vi "CRYScope-FFT.vi"(0 "Mode":u32(ring) items=["Time", "Spectrum"], 1 "Signal Path":i32(ring), 2 "Averages":i32=1 min=1, 3 "Time(sec)":dbl=0.05 min=0.05 max=10.0 step=0.05 format="%#.6p", 4 "Start":bool, 6 "Snap":bool, 7 "Hardware":string, 8 "Lin/Exp":i32(slide), 9 "Execution control":T6={"interactive"=TRUE, "displayed"=TRUE, "in a seq"=FALSE}, 10 "Manual":bool=TRUE, 11 "Calibration":string, 12 "Power/Complex":i32(slide)) -> (14 "Data cluster":T4, 16 "Avg. Complete":i32, 17 "Selected Signal Path":string, 18 "scope-fft setup Out":string="%#_6p", 19 "Canceled":bool)   [LabVIEW 2013]
uses:
  Typedef Control/CRYWaveform Cluster.ctl
  Typedef Control/CRYCalibration 2DCluster.ctl
  Typedef Control/CRYCalibration Cluster.ctl
  Typedef Control/CRYData Cluster.ctl
  Typedef Control/CRYHardware Channel Info.ctl
  SubVI/CRYMisc vis settings global.vi
  CRYMainGlobal.vi
  Calibration/SubVI/CRYCal Global.vi
  Task Sequence/CRYProject Run Control Global.vi
  <vilib>/Analysis/NI_AALPro.lvlib
  CRYSound.dll
panel:
  in  "Buf Cnt":i32
  in  "isMain":bool
  in  "Rcv Idx":u16
  in  "start_flg":u8
  in  "Remain Data":i32[](array[numeric])
  out "Asio OCI":u32
  in  "Device Name":string
  in  "ASIO_Inited":bool
  in  "Audio Driver":u16
  out "Max Level":dbl
  out "Load Test":bool
  out "Configure Data":string
  out "Set Configure":bool
  out "Calibration All Cluster":T1={"Calibration"={"Calibration Step Name"="", "Device"="", "Correction Curve Name"="", "Equalization Curve Name"="", "Sensitivity Curve Name"="", "Corr Folder and File"="", "EQ Folder and File"="", "Sens Folder and File"="", "Corr Step size"=0, "EQ Step size"=0, "Input"=FALSE, "Last Cal Date (sec)"=timestamp(0 s since 1904-01-01), "Cha Name"="", "Corr Curve Found"=FALSE, "EQ Curve Found"=FALSE, "Sens Curve Found"=FALSE, "Signal Type"="", "Calibrated Device"="", "Hz"=0}, "Corr Curve"={"Name"="", "Curve"=[], "X data"=1, "Y data"=1, "Z data"=1, "X axis"=0, "Y axis"=1, "Z axis"=1, "X unit"="", "Y unit"="", "Z unit"="deg.", "X dB ref"=1.0, "Y dB ref"=1.0, "Z dB ref"=1.0, "single val"=FALSE, "protected"=FALSE, "display X"=FALSE, "display Y"=TRUE, "display Z"=TRUE, "Test Info"="", "Step No."=0, "Plot Settings"={"Color"=0, "Interpolation"=0, "Point Style"=0, "Line Style"=0, "Point Color"=0, "Line Width"=0, "Bar Plot Style"=0, "Fill To"=0}, "AutoProtect"=FALSE}, "EQ Curve"={"Name"="", "Curve"=[], "X data"=1, "Y data"=1, "Z data"=1, "X axis"=0, "Y axis"=1, "Z axis"=1, "X unit"="Hz", "Y unit"="", "Z unit"="deg.", "X dB ref"=1.0, "Y dB ref"=1.0, "Z dB ref"=1.0, "single val"=FALSE, "protected"=FALSE, "display X"=TRUE, "display Y"=TRUE, "display Z"=TRUE, "Test Info"="", "Step No."=0, "Plot Settings"={"Color"=0, "Interpolation"=0, "Point Style"=0, "Line Style"=0, "Point Color"=0, "Line Width"=0, "Bar Plot Style"=0, "Fill To"=0}, "AutoProtect"=FALSE}, "Sens Curve"={"Name"="", "Curve"=[], "X data"=1, "Y data"=1, "Z data"=1, "X axis"=0, "Y axis"=1, "Z axis"=1, "X unit"="Hz", "Y unit"="", "Z unit"="deg.", "X dB ref"=1.0, "Y dB ref"=1.0, "Z dB ref"=1.0, "single val"=FALSE, "protected"=FALSE, "display X"=TRUE, "display Y"=TRUE, "display Z"=TRUE, "Test Info"="", "Step No."=0, "Plot Settings"={"Color"=0, "Interpolation"=0, "Point Style"=0, "Line Style"=0, "Point Color"=0, "Line Width"=0, "Bar Plot Style"=0, "Fill To"=0}, "AutoProtect"=FALSE}} {"Sens Curve"."Z data" items=["dB", "Lin"]; "Sens Curve"."X data" items=["dB", "Lin"]; "Sens Curve"."Y data" items=["dB", "Lin"]; "Sens Curve"."Z dB ref" format="%.1f"; "Sens Curve"."Z axis" items=["Log", "Lin"]; "Sens Curve"."X dB ref" format="%.1f"; "Sens Curve"."X axis" items=["Log", "Lin"]; "Sens Curve"."Y axis" items=["Log", "Lin"]; "Sens Curve"."Y dB ref" format="%.1f"; "Sens Curve"."Curve"."z" format="%.2f"; "Sens Curve"."Curve"."y" format="%.2f"; "Sens Curve"."Curve"."x" format="%.2f"; "EQ Curve"."Z data" items=["dB", "Lin"]; "EQ Curve"."X data" items=["dB", "Lin"]; "EQ Curve"."Y data" items=["dB", "Lin"]; "EQ Curve"."Z dB ref" format="%.1f"; "EQ Curve"."Z axis" items=["Log", "Lin"]; "EQ Curve"."X dB ref" format="%.1f"; "EQ Curve"."X axis" items=["Log", "Lin"]; "EQ Curve"."Y axis" items=["Log", "Lin"]; "EQ Curve"."Y dB ref" format="%.1f"; "EQ Curve"."Curve"."z" format="%.2f"; "EQ Curve"."Curve"."y" format="%.2f"; "EQ Curve"."Curve"."x" format="%.2f"; "Corr Curve"."Z data" items=["dB", "Lin"]; "Corr Curve"."X data" items=["dB", "Lin"]; "Corr Curve"."Y data" items=["dB", "Lin"]; "Corr Curve"."Z dB ref" format="%.1f"; "Corr Curve"."Z axis" items=["Log", "Lin"]; "Corr Curve"."X dB ref" format="%.1f"; "Corr Curve"."X axis" items=["Log", "Lin"]; "Corr Curve"."Y axis" items=["Log", "Lin"]; "Corr Curve"."Y dB ref" format="%.1f"; "Corr Curve"."Curve"."z" format="%.2f"; "Corr Curve"."Curve"."y" format="%.2f"; "Corr Curve"."Curve"."x" format="%.2f"; "Calibration"."EQ Step size" items=["R10", "R20", "R40", "R80", "User"]; "Calibration"."Corr Step size" items=["R10", "R20", "R40", "R80", "User"]}
  out "Est.Unit":string
  out "dB":dbl caption="Est.Level" format="%.3g"
  out "Cursor":bool
  out "initialized array":i32[](array[numeric])
  out "Menu":bool=TRUE
  out "StateOut":bool=TRUE
  out "VI nID":i32
  out "Title nID":i32
  in  "delta_Y":dbl
  in  "delta_X":dbl format="%#.3p"
  in  "delta_str":string
  out "rem buffer":i32[](array[numeric])
  out "dB Est.Level":dbl=33.979400086720375 format="%.2p"
  out "Channel In":u16
  in  "Waveform Cluster":T5={"Waveform"={"X0"=0.0, "dX"=0.0, "Y"=[]}, "X data"=1, "Y data"=1, "Y axis"=1, "X unit"="s", "Y unit"="s", "Y dB ref"=1.0, "display Y"=TRUE, "display X"=TRUE, "Overload?"=TRUE, "Test Info"="", "Step No."=0, "Name"="", "protected"=FALSE, "Sqc history"=[], "Signal Channel ID"=0, "Plot Settings"={"Color"=0, "Interpolation"=0, "Point Style"=0, "Line Style"=0, "Point Color"=0, "Line Width"=0, "Bar Plot Style"=0, "Fill To"=0}, "AutoProtect"=FALSE} {"Y dB ref" format="%.1f"; "Y axis" items=["Log", "Lin"]; "Y data" items=["dB", "Lin"]; "X data" items=["dB", "Lin"]}
  out "Triggered":bool
  out "AvgT":bool
  in  "Window":u16(ring) items=["None"=0, "Hanning"=1, "Hamming"=2, "Blackman-Harris"=3, "Exact Blackman"=4, "Blackman"=5, "Flat Top"=6, "4 Term B-Harris"=7, "7 Term B-Harris"=8, "Low Sidelobe"=9, "Blackman Nuttall"=11, "Triangle"=30, "Modified Bartlett-Hanning"=31, "Bohman"=32, "Parzen"=33, "Welch"=34, "Kaiser"=60, "Dolph-Chebyshev"=61, "Gaussian"=62]
  out "Spectrum graph":cluster{dbl, "df":dbl, "Spectrum":dbl[]}(graph)
  out "Buffer":u8(slide) scale=0.0..100.0
  out "Signal Graph":bool
  out "Averaging":bool
  out "Resolution":bool
  out "Input":bool
  out "Spectrum":bool
  out "Trigger":bool
  in  "taskID":u32
  out "Overload":bool
  in  "Slope":u32(slide) scale=0.0..1.0
  in  "Trigger Unit":u32(slide) scale=0.0..1.0
  out "Scale":bool
  in  "n points":i32=2048 caption="FFT lines" min=256 max=100000 step=256
  in  "Channels":u8=2
  out "Device In":u32
  in  "cont loop":bool=TRUE
  in  "Sensitivity":dbl=1.0 caption="V/unit" format="%.4f"
  in  "dB ref.":dbl=1.0 format="%.2f"
  in  "Y Unit":string
  in  "Y-axis":u16(ring) items=["dB", "Linear"]
  out "VMax In":dbl=10.0 format="%.3f"
  out "Bits":u32=16
  out "Sampling rate":u32=44100
  in  "close at end":bool
  out "THD":dbl max=10.0 format="%#_4p"
  in  "Harmonic":bool caption="Harmonic Cursor"
  in  "CalSpectrum":bool=TRUE caption="Calculate Spectrum"
  out "Hz":dbl caption="Est.Freq" format="%.1f"
  in  "Continue":bool
  in  "Correct":bool caption="Apply Correction"
  out "Real Time":u8(slide) scale=0.0..10.0
  out "Time graph":T7(graph)
  in  "dF(Hz)":dbl format="%#_6p"
  in  "dT(sec)":dbl format="%#_6p"
  in  "Spectral Lines":dbl min=256.0 format="%#_4p"
  in  "FreeRun":bool
  in  "Trigger Offset(sec)":dbl caption="Trigger Offset(s)" min=-0.05 max=0.05 format="%#_6p"
  in  "Trigger Level":dbl format="%#_5p"
  in  "Cancel":bool
  in  "Save":bool
  in  "OK":bool
  in  "A/M/M":i32(slide)
  in  "Trigger Path":u16(ring)
  in  "Weighting":u16(ring) items=["None", "A", "B", "C"]
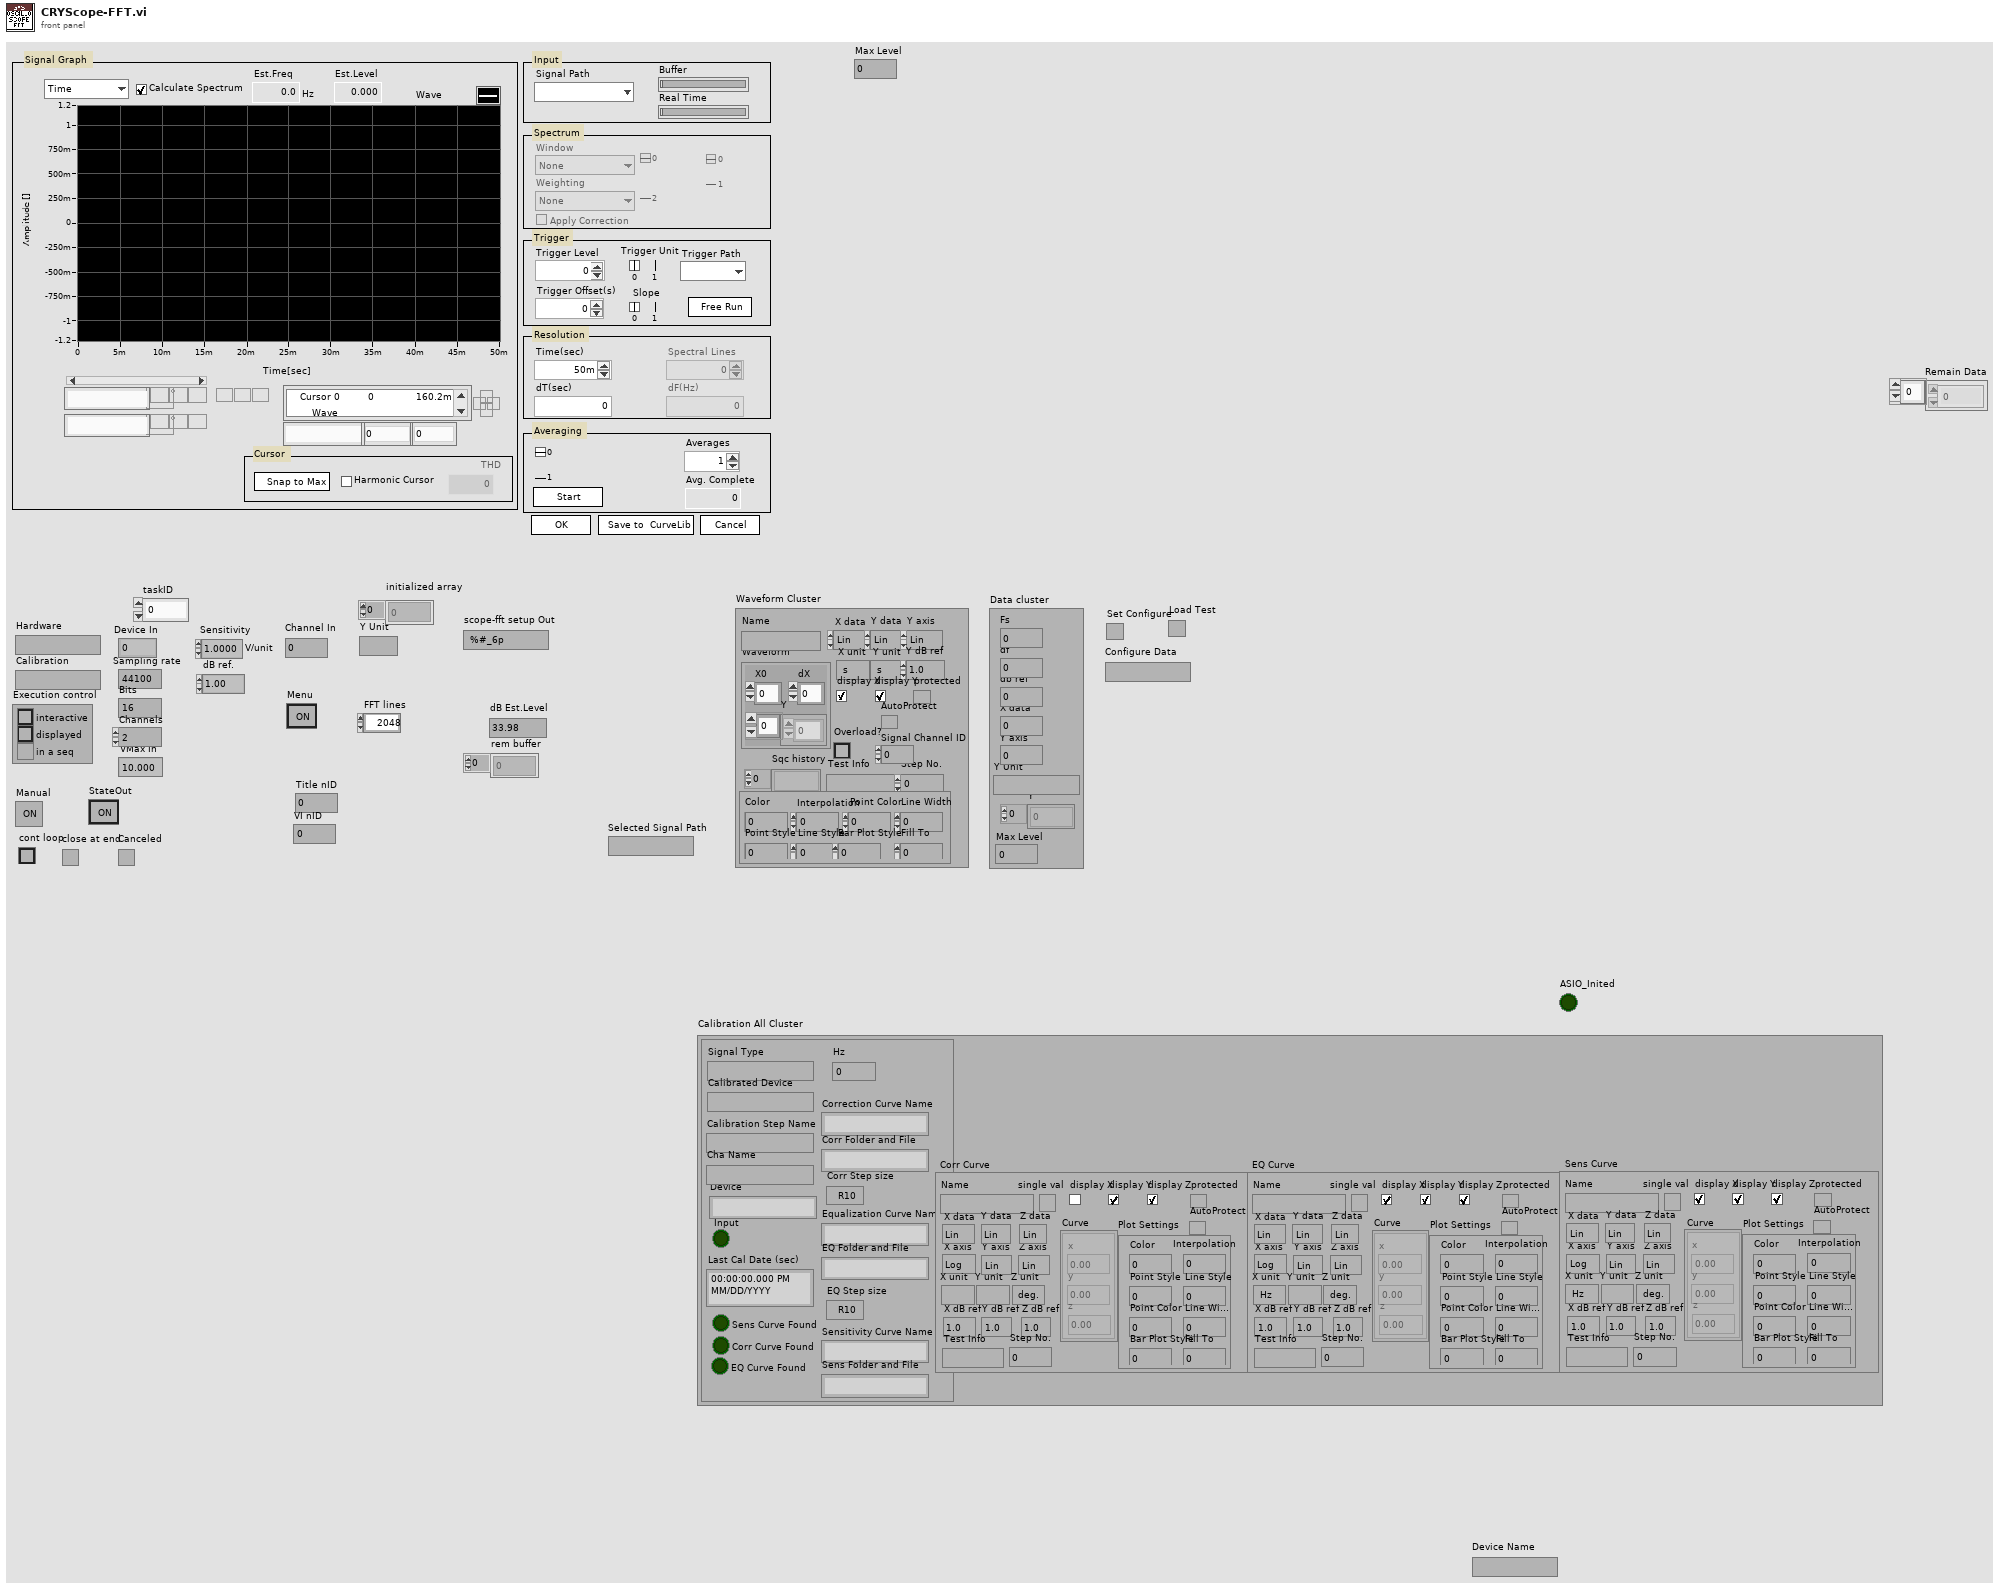
[diagram p1: front panel]
types:
  T1 = typedef "CRYCalibration 2DCluster.ctl" = cluster{"Calibration":T2, "Corr Curve":T3, "EQ Curve":T3, "Sens Curve":T3}
  T2 = typedef "CRYCalibration Cluster.ctl" = cluster{"Calibration Step Name":string, "Device":string, "Correction Curve Name":string, "Equalization Curve Name":string, "Sensitivity Curve Name":string, "Corr Folder and File":string, "EQ Folder and File":string, "Sens Folder and File":string, "Corr Step size":u16, "EQ Step size":u16, "Input":bool, "Last Cal Date (sec)":timestamp, "Cha Name":string, "Corr Curve Found":bool, "EQ Curve Found":bool, "Sens Curve Found":bool, "Signal Type":string, "Calibrated Device":string, "Hz":u32}
  T3 = typedef "CRYData Cluster.ctl" = cluster{"Name":string, "Curve":cluster{"x":dbl, "y":dbl, "z":dbl}[], "X data":u16, "Y data":u16, "Z data":u16, "X axis":u16, "Y axis":u16, "Z axis":u16, "X unit":string, "Y unit":string, "Z unit":string, "X dB ref":dbl, "Y dB ref":dbl, "Z dB ref":dbl, "single val":bool, "protected":bool, "display X":bool, "display Y":bool, "display Z":bool, "Test Info":string, "Step No.":i32, "Plot Settings":cluster{"Color":u32, "Interpolation":u8, "Point Style":u8, "Line Style":u8, "Point Color":u32, "Line Width":u8, "Bar Plot Style":u8, "Fill To":i16}, "AutoProtect":bool}
  T4 = cluster{"Fs":dbl, "df":dbl, "db ref":dbl, "X data":u16, "Y axis":u16, "Y Unit":string, "Y":dbl[], "Max Level":dbl}
  T5 = typedef "CRYWaveform Cluster.ctl" = cluster{"Waveform":cluster{"X0":dbl, "dX":dbl, "Y":sgl[]}, "X data":u16, "Y data":u16, "Y axis":u16, "X unit":string, "Y unit":string, "Y dB ref":dbl, "display Y":bool, "display X":bool, "Overload?":bool, "Test Info":string, "Step No.":i32, "Name":string, "protected":bool, "Sqc history":string[], "Signal Channel ID":i32, "Plot Settings":cluster{"Color":u32, "Interpolation":u8, "Point Style":u8, "Line Style":u8, "Point Color":u32, "Line Width":u8, "Bar Plot Style":u8, "Fill To":i16}, "AutoProtect":bool}
  T6 = cluster{"interactive":bool, "displayed":bool, "in a seq":bool}
  T7 = cluster{dbl, "dT(sec)":dbl, "Triggered signal":dbl[]}
  T8 = cluster{"window":i32, "n avgs":i32, "lin/exp avg":i32, "pwr/cplx avg":i32, "time (ms)":dbl, "fft lines":i32, "scope/fft mode":i32, "channel":i32, "trig. channel":i32, "Applay Correction":bool, "Time Display":string, "Freq. Weighting":string, "Ave/Max/Min":u16, "Trigger Level":dbl, "Trigger Unit":u16, "Trigger Time Offset":dbl, "Trigger Slope":u16, "Trigger/Free Run":bool, "continuous":bool, "Spectrum Display":string, "Calc FFT":bool, "Y-axis":string, "Channel String":string}
  T9 = enum32{"Invalid", "Default", "Floating", "Floating/Auto-Hide", "Modal"}
  T10 = cluster{"Weighting":u16, "Signal Path":i32, "Y-axis":u16, "Time(sec)":dbl, "Mode":u32, "Power/Complex":i32, "Harmonic":bool, "Trigger Level":dbl, "n points":i32, "Lin/Exp":i32, "Trigger Offset(sec)":dbl, "Trigger Unit":u32, "Averages":i32, "Start":bool, "Spectral Lines":dbl, "A/M/M":i32, "FreeRun":bool}
  T11 = typedef "CRYCalibration All Cluster.ctl" = cluster{"Calibration 2D":T1[], "Help":string, "Tab Value":i32, "Input Signal Type":string, "Output Signal Type":string}
  T12 = typedef "CRYScope-FFT.ctl" = cluster{"window":i32, "n avgs":i32, "lin/exp avg":i32, "pwr/cplx avg":i32, "time (ms)":dbl, "fft lines":i32, "scope/fft mode":i32, "channel":i32, "trig. channel":i32, "Applay Correction":bool, "Time Display":string, "Freq. Weighting":string, "Ave/Max/Min":u16, "Trigger Level":dbl, "Trigger Unit":u16, "Trigger Time Offset":dbl, "Trigger Slope":u16, "Trigger/Free Run":bool, "continuous":bool, "Spectrum Display":string, "Calc FFT":bool, "Y-axis":string, "Signal Type":string}
  T13 = typedef "CRYHardware Channel Info.ctl" = cluster{"ID":i32, "Name":string, "Digital":bool, "Input":bool, "Device Name":string, "Hardware Ch ID":u8, "Vmax (V)":dbl, "Latency (samples)":dbl, "Sampling Rate (Hz)":u32, "Bit Depth":u32, "Anti-aliasing Factor (%fs)":sgl, "DAQmx Channel":tag, "term config":i32, "Coupling":i32, "IEPE en":bool, "ASIOChannel Name":string, "Audio Driver":u16, "ASIOChannel Index":u8}
  T14 = enum32{"English", "Chinese", "Korean", "Japanese", "Russian", "Chinese traditional"}
  T15 = enum32{"Vrms", "Vpk", "Vrms^2", "Vpk^2", "Vrms/rtHz", "Vpk/rtHz", "Vrms^2/Hz", "Vpk^2/Hz"}
  T16 = cluster{"acquire":bool, "halt acq":bool, "cal factor":dbl, "n avgd":i32, "db-pr factor":dbl, "points":i32, "buffers":i32, "points chg":bool, "db ref":dbl, "df":dbl, "window constants":cluster{"eq noise BW":dbl, "coherent gain":dbl}, "cursor index":i32, "cursor x":dbl, "trig level":i32, "est freq":dbl, "est power":dbl, "update":bool, "autoscale":bool, "avg. complete":i32, "prebuffer":i32, "nextbuffer":i32, "addbuffs":i32, "Y-axis chg":bool, "Weight":cluster{dbl, dbl}[]}
  T17 = typedef "CRYStimulus Test Infor Cluster.ctl" = cluster{"Stimulus Type":string, "Signal Type":string, "In/Out":bool, "FAPS":cluster{"freq":dbl, "ampl":dbl, "cycles":dbl, "samples":i32}[], "Sampling Rate":dbl, "Samples":i32, "Analysis Param":string, "Resolution":u16, "Steps":u32, "Analysis Value":dbl[], "Diff Freq":dbl, "FStart":dbl, "FStop":dbl, "Calibration Param":string, "Anti Alias":dbl, "Level Out1":dbl, "Level Out2":dbl, "EQ":bool}
  T18 = cluster{"Name":string, "Color":u32, "Style":u8, "Point Style":u8, "Name Visible":bool, "Allow Drag":bool, "Lock Style":u32, "Plot":u32, "Index":i32, "Position":cluster{"X":dbl, "Y":dbl}}[]
  T19 = cluster{"Cursor Name":string, "Cursor Color":u32, "Cursor Style":u8, "Cursor Point Style":u8, "Cursor Name Visible":bool, "Allow Drag":bool, "Cursor Locked":u32, "Cursor Plot":u32, "Cursor Index":i32, "Cursor Position":cluster{"Cursor X":dbl, "Cursor Y":dbl}}[]
  T20 = typedef "LVCursorListTypeDef.ctl" = cluster{"Name":string, "Color":u32, "Style":u8, "Point Style":u8, "Name Visible":bool, "Allow Drag":bool, "Cursor Mode":u32, "Plot":i32, "Index":i32, "Position":cluster{"X":dbl, "Y":dbl}, "X Scale":u32, "Y Scale":u32, "Watch Plots":i32[], "Watch All Plots":bool, "Plot Area":i32, "Label Offset":cluster{"X":dbl, "Y":dbl}}[]
  T21 = cluster{"Name":string, "Color":u32, "Style":u8, "Point Style":u8, "Name Visible":bool, "Allow Drag":bool, "Cursor Mode":u32, "Plot":i32, "Index":i32, "Position":cluster{"X":dbl, "Y":dbl}, "X Scale":u32, "Y Scale":u32, "Watch Plots":i32[], "Watch All Plots":bool, "Plot Area":i32, "Label Offset":cluster{"X":dbl, "Y":dbl}}
  T22 = cluster{"Fs":dbl, "df":dbl, "db ref":dbl, "X data":u16, "Y data":u16, "Y Unit":string, "Y":dbl[], "Max Level":dbl}
  T23 = cluster{"Rcv Idx":i32, "Chn Idx":i32, "Data":i32[], "bufCount":i32}[]
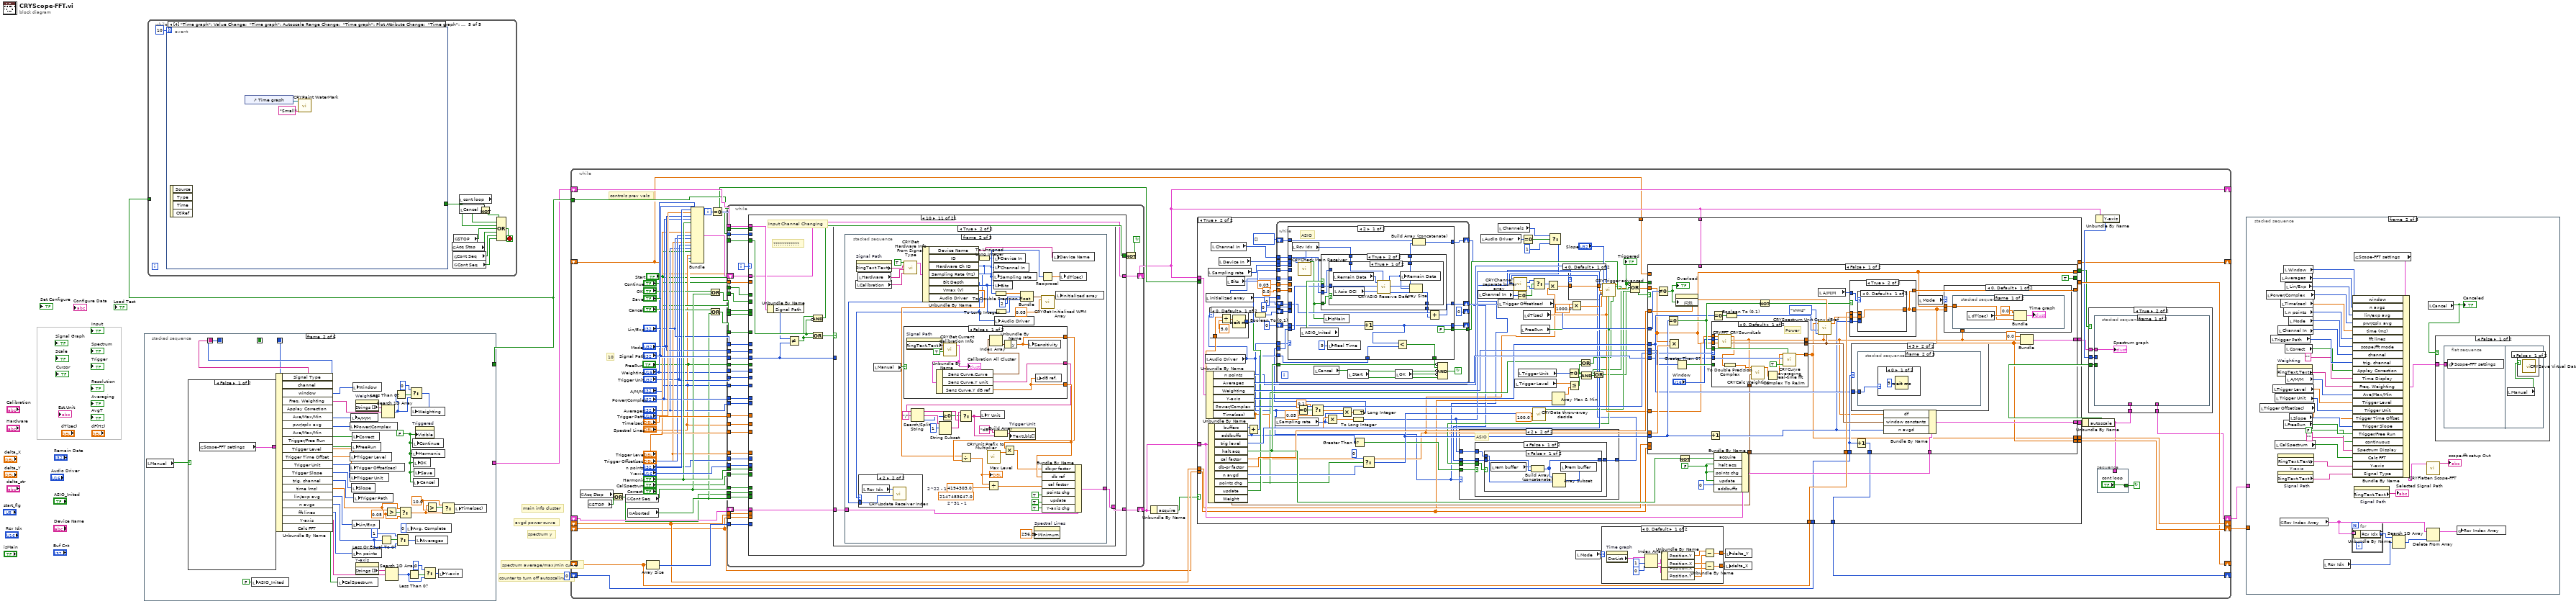
[diagram p0: block diagram]
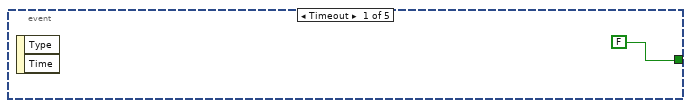
[diagram p2: hidden frame]
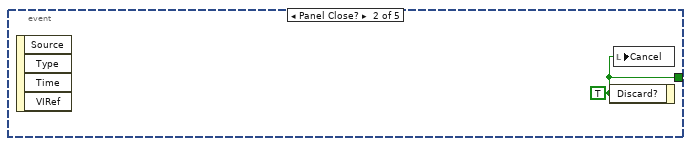
[diagram p3: hidden frame]
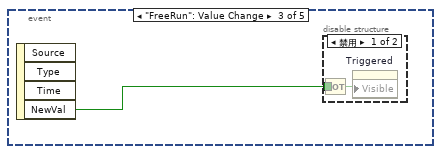
[diagram p4: hidden frame]
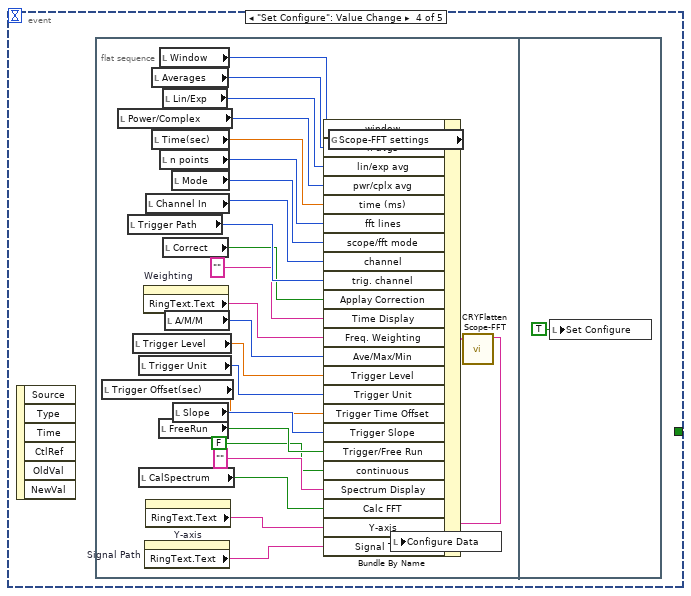
[diagram p6: hidden frame]
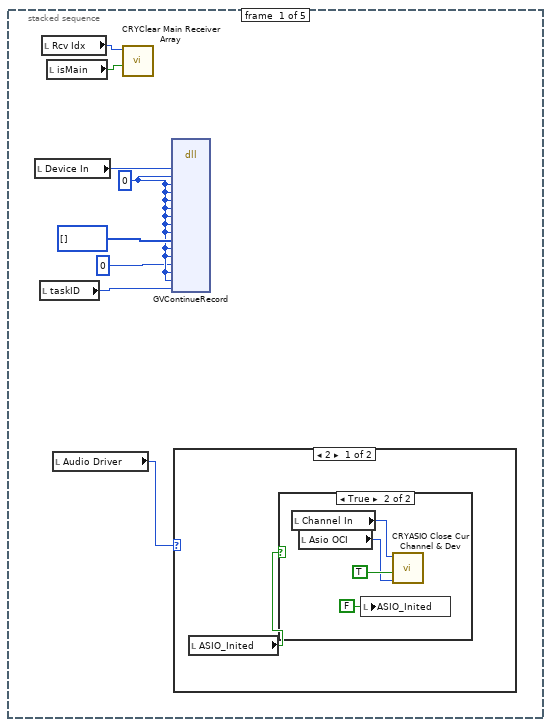
[diagram p7: hidden frame]
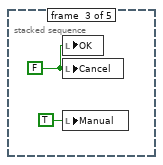
[diagram p12: hidden frame]
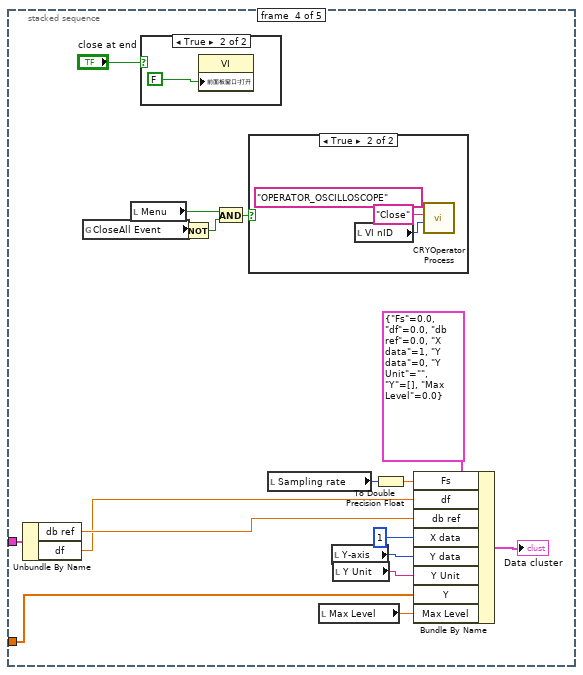
[diagram p13: hidden frame]
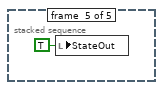
[diagram p16: hidden frame]
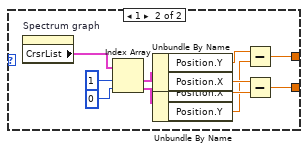
[diagram p17: hidden frame]
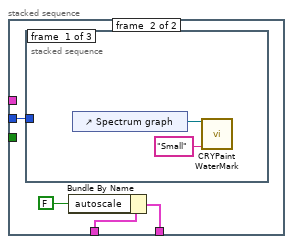
[diagram p19: hidden frame]
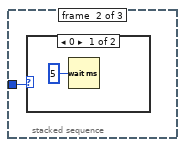
[diagram p20: hidden frame]
diagram:
  # "counter to turn off autoscaling"
  # "spectrum average/max/min curve"
  # "main info cluster"
  # "spectrum y"
  # "avgd power curve"
  n1 = stacked-sequence {
    seq-local: [_ w59 _ _ _ _] -> [_ _ _ w95 _ _]
    seq-local: [_ _ w81 _ _ _] -> [_ _ _ _ _ _]
    seq-local: [_ w65 _ _ _ _] -> [_ _ _ _ _ _]
    seq-local: [_ w67 _ _ _ _] -> [_ _ _ _ w109 _]
    tunnel: [_ _ w82 _ _ _] -> w3
    tunnel: [_ _ _ _ _ w180] -> w2
    frame #0 {
      n2 = global read "CRYMisc vis settings global.vi" "Menu?"() -> (w14:bool)
      "Menu" <- w14
      n3 = call "CRYMake Receiver Index.vi"() -> ("Receiver_Index"=w6:i32)  [unwired: 11 in]
      n4 = local write "Set Configure"(FALSE ("Set Configure")) -> ()
      n5 = local write "Rcv Idx"(w6) -> ()
      n6 = case shown="False" w14 {
        tunnel: [w19 w28] -> w13
        tunnel: "Oscilloscope-FFT" ("Kind") -> [w18 w23]
        tunnel: [w17 w21] -> w7
        frame False {
          n7 = control-ref of="This VI"() -> (w16:refnum<vi>)
          n8 = call "CRYSet Scope-FFT Front Panel.vi"("Vi Ref in"=w16) -> ()  [unwired: 10 in, 1 out]
          n9 = call "CRYGet Window Title Message.vi"("No"=0 ("Error No"), "Kind"=w18) -> ("Multibyte String"=w19:string)  [unwired: 4 in, 5 out]
          n10 = local read "Calibration"() -> (w17:string)
        }
        frame True {
          n11 = global read "CRYMisc vis settings global.vi" "scope-fft mode"() -> (w25:u32)
          n12 = global read "CRYMisc vis settings global.vi" "Execution control"() -> (w31:T6)
          n13 = call "CRYGet Current HC Steps.vi"() -> ("Calibration setup flattened Out"=w21:string, "Hardware setup flattened Out"=w22:string)  [unwired: 10 out]
          n14 = global read "CRYMisc vis settings global.vi" "Temp Title nID"() -> (w30:i32)
          "Title nID" <- w30
          n15 = global read "CRYMisc vis settings global.vi" "Temp VI nID"() -> (→"VI nID":i32)
          n16 = call "CRYGet Window Title Message.vi"("No"=w25, "Kind"=w23) -> ("Multibyte String"=w24:string)  [unwired: 4 in, 5 out]
          n17 = global read "CRYMisc vis settings global.vi" "Manual"() -> (w32:bool)
          n18 = local write "Calibration"(w21) -> ()
          n19 = local write "Hardware"(w22) -> ()
          n20 = local write "Execution control"(w31) -> ()
          n21 = local write "Manual"(w32) -> ()
          n22 = local write "Mode"(w25) -> ()
          n23 = Number To Decimal String(number=w30) -> (decimal integer string=w27:string)  [unwired: 1 in]
          n24 = Concatenate Strings(w24, "-" ("string"), w27) -> (w28:string)
        }
      }
      n25 = property class="VI"("Front Panel.Title"=w13) -> ()  [unwired: 2 in, 2 out]
      n26 = call "CRYUnflatten Calibration 2D.vi"("Flattened Calibration"=w7) -> ("Calibration Step Out"=w8:T11)  [unwired: 8 in, 2 out]
      n27 = call "CRYGet Weight Name Array.vi"() -> ("Weighting Names"=w11:string[])  [unwired: 11 in]
      n28 = call "CRYGet Calibrated Device Name.vi"("Calibration"=w8) -> ("I_Signal Type Out"=w9:string[])  [unwired: 7 in, 7 out]
      n29 = property on="Weighting" class="Ring (strict)"("Strings []"=w11) -> ()  [unwired: 2 in, 2 out]
      n30 = property on="Trigger Path" class="Ring (strict)"("Strings []"=w9) -> ()  [unwired: 2 in, 2 out]
      n31 = property on="Signal Path" class="Ring (strict)"("Strings []"=w9) -> ()  [unwired: 2 in, 2 out]
      "StateOut" <- FALSE ("StateOut")
    }
    frame #1 {
      w41 = 10.0 ("y")
      w44 = 0.05 ("y")
      w74 = FALSE ("Start")
      n32 = local read "Manual"() -> (w73:bool)
      n33 = case shown="False" w73 {
        tunnel: [w76 T8 {"window"=0, "n avgs"=1, "lin/exp avg"=0, "pwr/cplx avg"=0, "time (ms)"=0.05, "fft lines"=2048, "scope/fft mode"=0, "channel"=0, "trig. channel"=0, "Applay Correction"=FALSE, "Time Display"="%#_6p", "Freq. Weighting"="%.1f", "Ave/Max/Min"=0, "Trigger Level"=0.0, "Trigger Unit"=2, "Trigger Time Offset"=0.01, "Trigger Slope"=0, "Trigger/Free Run"=TRUE, "continuous"=FALSE, "Spectrum Display"="%#_6p", "Calc FFT"=FALSE, "Y-axis"="None", "Channel String"="Left"} ("Scope-FFT settings")] -> w75
        frame False {
          n34 = global read "CRYMisc vis settings global.vi" "Scope-FFT settings"() -> (w76:T12)
        }
        frame True {
        }
      }
      n35 = local write "ASIO_Inited"(FALSE ("ASIO_Inited")) -> ()
      n36 = Unbundle By Name(w75) -> ("Signal Type"=w67:string, "channel"=w65:i32, "window"=w66:i32, "Freq. Weighting"=w63:string, "Applay Correction"=w54:bool, "Ave/Max/Min"=w62:u16, "pwr/cplx avg"=w61:i32, "Trigger/Free Run"=w72:bool, "Trigger Level"=w71:dbl, "Trigger Time Offset"=w70:dbl, "Trigger Unit"=w69:u16, "Trigger Slope"=w68:u16, "trig. channel"=w60:i32, "time (ms)"=w43:dbl, "lin/exp avg"=w59:i32, "n avgs"=w36:i32, "fft lines"=w58:i32, "Y-axis"=w56:string, "Calc FFT"=w55:bool)  [unwired: 1 out]
      n37 = local write "CalSpectrum"(w55) -> ()
      n38 = local write "Power/Complex"(w61) -> ()
      n39 = local write "Trigger Offset(sec)"(w70) -> ()
      n40 = local write "Trigger Level"(w71) -> ()
      n41 = local write "Trigger Unit"(w69) -> ()
      n42 = local write "A/M/M"(w62) -> ()
      n43 = local write "FreeRun"(w72) -> ()
      n44 = local write "Slope"(w68) -> ()
      n45 = local write "Correct"(w54) -> ()
      n46 = local write "Lin/Exp"(w59) -> ()
      n47 = local write "n points"(w58) -> ()
      n48 = local write "Window"(w66) -> ()
      n49 = local write "Trigger Path"(w60) -> ()
      n50 = property on="Weighting" class="Ring (strict)"() -> ("Strings []"=w64:string[])  [unwired: 2 in, 2 out]
      n51 = property on="Y-axis" class="Ring (strict)"() -> ("Strings []"=w57:string[])  [unwired: 2 in, 2 out]
      n52 = Less Or Equal To 0?(x=w36) -> (x <= 0?=w37:bool)
      n53 = Search 1D Array(1D array=w64, element=w63) -> (index of element=w47:i32)  [unwired: 1 out]
      n54 = Greater?(x=w43, y=w44) -> (0:w45:bool)
      n55 = Search 1D Array(1D array=w57, element=w56) -> (index of element=w50:i32)  [unwired: 1 out]
      n56 = Less Than 0?(x=w47) -> (x < 0?=w49:bool)
      n57 = Select(t=1 ("n avgs"), s=w37, f=w36) -> (s? t:f=w34:i32)
      n58 = Select(t=w43, s=w45, f=w44) -> (s? t:f=w40:dbl)
      n59 = local write "Avg. Complete"(0 ("Avg. Complete")) -> ()
      n60 = Less Than 0?(x=w50) -> (x < 0?=w53:bool)
      n61 = Select(t=0 ("index of element"), s=w49, f=w47) -> (s? t:f=w46:i32)
      n62 = local write "Weighting"(w46) -> ()
      n63 = local write "Harmonic"(w74) -> ()
      n64 = local write "Continue"(w74) -> ()
      n65 = local write "Cancel"(w74) -> ()
      n66 = local write "OK"(w74) -> ()
      n67 = local write "Save"(w74) -> ()
      n68 = property on="Triggered" class="Bool (strict)"("Visible"=w74) -> ()  [unwired: 2 in, 2 out]
      n69 = local write "Averages"(w34) -> ()
      n70 = Select(t=0 ("index of element"), s=w53, f=w50) -> (s? t:f=w51:i32)
      n71 = Greater?(x=w40, y=w41) -> (0:w42:bool)
      n72 = local write "Y-axis"(w51) -> ()
      n73 = Select(t=w41, s=w42, f=w40) -> (s? t:f=w39:dbl)
      n74 = local write "Time(sec)"(w39) -> ()
    }
    frame #2 {
      n75 = control-ref of="This VI"() -> (w79:refnum<vi>)
      n76 = Unbundle By Name("Execution control") -> ("in a seq"=w81:bool, "interactive"=w88:bool, "displayed"=w83:bool)
      n77 = property class="VI"() -> ("前面板窗口:打开"=w85:bool)  [unwired: 2 in, 2 out]
      n78 = property class="VI"(reference=w79, "FP.Behavior"=T9."Floating" ("Front Panel Window:Behavior")) -> ()  [unwired: 1 in, 2 out]
      n79 = property on="Start" class="Bool (strict)"("Value"=TRUE ("Start")) -> ()  [unwired: 2 in, 2 out]
      n80 = Or(x=w88, y=w83) -> (x .or. y?=w86:bool)
      n81 = Not(x=w81) -> (.not. x?=w82:bool)
      n82 = Compound Arithmetic op=AND(w86, invert w85) -> (w87:bool)
      n83 = case shown="True" w86 {
        tunnel: w86 -> [_ w89]
        tunnel: w87 -> [_ _]
        frame False {
        }
        frame True {
          n84 = stacked-sequence {
            tunnel: w89 -> [w90 _ _]
            frame #0 {
              n85 = property class="VI"("前面板窗口:打开"=w90) -> ()  [unwired: 2 in, 2 out]
            }
            frame #1 {
              n86 = Wait (ms)(milliseconds to wait=u32 150) -> ()  [unwired: 1 out]
            }
            frame #2 {
            }
          }
        }
      }
      n87 = local write "close at end"(w87) -> ()
    }
    frame #3 {
      # "weight"
      n88 = local write "start_flg"(u8 1 ("start_flg")) -> ()
      n89 = case shown="0" w95 {
        tunnel: [w103 w107] -> w94
        frame Default {
          n90 = call "CRYGet Error Message.vi"("Error No"=1, "Kind"="Oscilloscope-FFT Sub") -> ("Unicode Message Sub"=w103:string[])  [unwired: 4 in, 5 out]
        }
        frame 0 {
          n91 = call "CRYGet Error Message.vi"("Error No"=0, "Kind"="Oscilloscope-FFT Sub") -> ("Unicode Message Sub"=w107:string[])  [unwired: 4 in, 5 out]
        }
      }
      n92 = case shown="1" w95 {
        frame 0, Default {
          n93 = property on="Avg. Complete" class="DigNum (strict)"("Visible"=TRUE) -> ()  [unwired: 2 in, 2 out]
          n94 = property on="AvgT" class="Bool (strict)"("Visible"=FALSE ("AvgT")) -> ()  [unwired: 2 in, 2 out]
        }
        frame 1 {
          n95 = property on="Avg. Complete" class="DigNum (strict)"("Visible"=FALSE) -> ()  [unwired: 2 in, 2 out]
          n96 = property on="AvgT" class="Bool (strict)"("Visible"=TRUE ("AvgT")) -> ()  [unwired: 2 in, 2 out]
          n97 = property on="AvgT" class="Bool (strict)"("Value"=TRUE ("AvgT")) -> ()  [unwired: 2 in, 2 out]
        }
      }
      n98 = for {
        tunnel: w94 -> [w97] mode=indexing
        tunnel: [w96] -> w93 mode=indexing
        n99 = call "CRYConvert Unicode to ASCII.vi"("Unicode"=w97) -> ("ASCII"=w96:string)  [unwired: 4 in]
      }
      n100 = property on="Start" class="Bool (strict)"("Strings [4]"=w93) -> ()  [unwired: 2 in, 2 out]
    }
    frame #4 {
      w124 = u8 2 ("Write Attribute")
      n101 = property on="Spectrum graph" class="WFGraph (strict)"("Y标尺.标尺调节"=w124) -> ()  [unwired: 2 in, 2 out]
      n102 = property on="Time graph" class="WFGraph (strict)"("XScale.ScaleFit"=w124) -> ()  [unwired: 2 in, 2 out]
      n103 = case shown="False" "Manual" {
        tunnel: [w128 w143] -> w111
        tunnel: [w126 w142] -> w112
        tunnel: w109 -> [_ w137]
        frame True {
          w128 = u32 44100 ("Sampling rate")
          w126 = u32 16 ("Bit Depth")
          (unwired) T13[] [{"ID"=2, "Name"="Left", "Digital"=FALSE, "Input"=TRUE, "Device Name"="Card", "Hardware Ch ID"=0, "Vmax (V)"=10.0, "Latency (samples)"=67.0, "Sampling Rate (Hz)"=44100, "Bit Depth"=16, "Anti-aliasing Factor (%fs)"=44100.0, "DAQmx Channel"="", "term config"=0, "Coupling"=0, "IEPE en"=FALSE, "ASIOChannel Name"="", "Audio Driver"=0, "ASIOChannel Index"=0}, {"ID"=2, "Name"="Right", "Digital"=FALSE, "Input"=TRUE, "Device Name"="Card", "Hardware Ch ID"=1, "Vmax (V)"=10.0, "Latency (samples)"=67.0, "Sampling Rate (Hz)"=44100, "Bit Depth"=16, "Anti-aliasing Factor (%fs)"=44100.0, "DAQmx Channel"="", "term config"=0, "Coupling"=0, "IEPE en"=FALSE, "ASIOChannel Name"="", "Audio Driver"=0, "ASIOChannel Index"=0}]  # I_channel Info Out
          n104 = global write "CRYMainGlobal.vi" "STOP"(FALSE ("STOP")) -> ()
          "Device In" <- u32 2 ("Device In")
          "Bits" <- w126
          "VMax In" <- 10.0 ("VMax In")
          "Sampling rate" <- w128
          "Channel In" <- u16 0 ("Channel In")
        }
        frame False {
          n105 = global read "CRYCal Global.vi" "Calibrate"() -> (w139:bool)
          n106 = local read "Calibration"() -> (w141:string)
          n107 = local read "Hardware"() -> (w140:string)
          n108 = case shown="True" w139 {
            tunnel: w137 -> [w153 _]
            tunnel: [w156 w171] -> w136
            tunnel: w140 -> [w155 w173]
            tunnel: w141 -> [w154 w172]
            tunnel: [w150 w170] -> w138
            frame False {
              n109 = call "CRYGet Hardware Info From Signal Type.vi"("Calibration In"=w154, "Hardware In"=w155, "Signal Type"=w153, "In/Out?"=TRUE) -> ("Exist?"=w158:bool, "Channel Info Out"=w157:T13)  [unwired: 5 in, 1 out]
              n110 = property on="Signal Path" class="Ring (strict)"() -> ("Strings []"=w152:string[])  [unwired: 2 in, 2 out]
              n111 = case shown="False" w158 {
                tunnel: w157 -> [_ w166]
                tunnel: [w161 w166] -> w156
                tunnel: w155 -> [w164 _]
                tunnel: w154 -> [w163 _]
                tunnel: w153 -> [_ w165]
                tunnel: [w160 w165] -> w151
                frame False {
                  w160 = "Direct In 1" ("Signal Type")
                  n112 = call "CRYGet Hardware Info From Signal Type.vi"("Calibration In"=w163, "Hardware In"=w164, "Signal Type"=w160, "In/Out?"=TRUE) -> ("Channel Info Out"=w161:T13)  [unwired: 5 in, 2 out]
                }
                frame True {
                }
              }
              n113 = Search 1D Array(1D array=w152, element=w151) -> (index of element=w150:i32)  [unwired: 1 in]
            }
            frame True {
              n114 = global read "CRYCal Global.vi" "Signal Type In"() -> (w170:u16)
              n115 = property on="Signal Path" class="Ring (strict)"() -> ("Strings []"=w169:string[])  [unwired: 2 in, 2 out]
              n116 = Index Array(array=w169, index=w170) -> (element=w167:string)
              n117 = call "CRYGet Hardware Info From Signal Type.vi"("Calibration In"=w172, "Hardware In"=w173, "Signal Type"=w167, "In/Out?"=TRUE) -> ("Channel Info Out"=w171:T13)  [unwired: 5 in, 2 out]
            }
          }
          n118 = local write "Signal Path"(w138) -> ()
          n119 = Unbundle By Name(w136) -> ("ID"=w145:i32, "Vmax (V)"=w144:dbl, "Sampling Rate (Hz)"=w143:u32, "Bit Depth"=w142:u32, "Hardware Ch ID"=w132:u8, "Audio Driver"=w133:u16, "Device Name"=w134:string)
          n120 = case shown="2" w133 {
            tunnel: w132 -> [_ w148]
            frame 0, Default {
              n121 = local read "Rcv Idx"() -> (w147:u16)
              n122 = call "CRYUpdate Receiver Index.vi"("Chn Idx"=-1, "Receiver_Index"=w147) -> ()  [unwired: 9 in]
            }
            frame 2 {
              n123 = local read "Rcv Idx"() -> (w149:u16)
              n124 = call "CRYUpdate Receiver Index.vi"("Chn Idx"=w148, "Receiver_Index"=w149) -> ()  [unwired: 9 in]
            }
          }
          n125 = To Unsigned Long Integer(number=w145) -> (unsigned 32bit integer=w135:u32)
          n126 = local write "Device Name"(w134) -> ()
          n127 = local write "Audio Driver"(w133) -> ()
          n128 = local write "Sampling rate"(w143) -> ()
          n129 = local write "VMax In"(w144) -> ()
          n130 = local write "Channel In"(w132) -> ()
          n131 = local write "Device In"(w135) -> ()
          n132 = local write "Bits"(w142) -> ()
        }
      }
      n133 = local read "Time(sec)"() -> (w122:dbl)
      n134 = Divide(x=w111, y=2.0) -> (x/y=w120:dbl)
      n135 = Multiply(x=w122, y=w120) -> (x*y=w119:dbl)
      n136 = Reciprocal(x=w111) -> (1/x=w123:dbl)
      n137 = To Double Precision Float(number=w111) -> (double precision float=w117:dbl)
      n138 = To Long Integer(number=w112) -> (32bit integer=w116:i32)
      n139 = Round Toward -Infinity(1:w119) -> (0:w118:dbl)
      n140 = local write "dT(sec)"(w123) -> ()
      n141 = local write "Spectral Lines"(w118) -> ()
      n142 = Bundle(w117, "32bit integer"=2, w116) -> (w114:cluster{dbl, "32bit integer":i32, i32})  [unwired: 1 in]
      n143 = call "CRYGet Initialized WFM Array.vi"("Sound Format"=w114, "Time(s)"=0.05) -> ("initialized array"=→"initialized array":i32[])  [unwired: 8 in, 5 out]
    }
    frame #5 {
      n144 = global read "CRYMainGlobal.vi" "Language"() -> (w176:T14)
      n145 = case shown="\"Chinese\"" w176 {
        tunnel: ["D\u0000e\u0000l\u0000t\u0000a\u0000" ("delta_str") "î]<P" ("Unicode")] -> w175
        frame "English", Default {
        }
        frame "Chinese" {
        }
      }
      n146 = local write "Load Test"(TRUE ("Load Test")) -> ()
      n147 = local write "cont loop"(TRUE ("cont loop")) -> ()
      n148 = call "CRYConvert Unicode to ASCII.vi"("Unicode"=w175) -> ("ASCII"=w174:string)  [unwired: 4 in]
      n149 = local write "delta_str"(w174) -> ()
      n150 = local read "FreeRun"() -> (w179:bool)
      n151 = Not(x=w179) -> (.not. x?=w178:bool)
      n152 = Bundle By Name(cluster=T10 {"Weighting"=0, "Signal Path"=65535, "Y-axis"=0, "Time(sec)"=-1.0, "Mode"=0, "Power/Complex"=0, "Harmonic"=FALSE, "Trigger Level"=0.0, "n points"=0, "Lin/Exp"=0, "Trigger Offset(sec)"=0.0, "Trigger Unit"=0, "Averages"=0, "Start"=FALSE, "Spectral Lines"=0.0, "A/M/M"=0, "FreeRun"=TRUE}, "FreeRun"=w178) -> (w180:T10)
    }
  }
  n153 = while {
    tunnel: w3 -> [_]
    stop <- w191 stop-if-true
    n154 = event shown="[4] \"Time graph\": Value Change;  \"Time graph\": Autoscale Range Change;  \"Time graph\": Plot Attribute Change;  \"Time graph\": Scale Range Change" {
      selector: _ -> [_ _ _ _ _]
      dyn-events: _ -> [_ _ _ _ _]
      timeout: 10 -> [_ _ _ _ _]
      tunnel: [FALSE ("Discard?") w196 _ _ _] -> w193
      event Timeout {
        n155 = event-data() -> ()  [unwired: 3 out]
      }
      event Panel Close? {
        w196 = TRUE ("Discard?")
        n156 = event-data() -> ()  [unwired: 5 out]
        n157 = event-data("Discard?"=w196) -> ()  [unwired: 1 in, 1 out]
        n158 = local write "Cancel"(w196) -> ()
      }
      event "FreeRun": Value Change {
        n159 = event-data() -> ("NewVal"=w197:bool)  [unwired: 4 out]
        n160 = disable-structure shown="禁用" {
          disable-tunnel: w197 -> [w199 _]
          frame Disabled {
            n161 = Not(x=w199) -> (.not. x?=w198:bool)
            n162 = property on="Triggered" class="Bool (strict)"("Visible"=w198) -> ()  [unwired: 2 in, 2 out]
          }
          frame Enabled {
          }
        }
      }
      event "Set Configure": Value Change {
        n163 = event-data() -> ()  [unwired: 7 out]
        n164 = flat-sequence {
          frame #0 {
            n165 = local read "Trigger Offset(sec)"() -> (w213:dbl)
            n166 = local read "Power/Complex"() -> (w223:i32)
            n167 = local read "Trigger Path"() -> (w218:u16)
            n168 = local read "Trigger Level"() -> (w212:dbl)
            n169 = local read "Trigger Unit"() -> (w214:u32)
            n170 = local read "CalSpectrum"() -> (w210:bool)
            n171 = property on="Weighting" class="Ring (strict)"() -> ("RingText.Text"=w204:string)  [unwired: 2 in, 2 out]
            n172 = property on="Signal Path" class="Ring (strict)"() -> ("RingText.Text"=w205:string)  [unwired: 2 in, 2 out]
            n173 = local read "Channel In"() -> (w206:u16)
            n174 = property on="Y-axis" class="Ring (strict)"() -> ("RingText.Text"=w202:string)  [unwired: 2 in, 2 out]
            n175 = local read "Averages"() -> (w221:i32)
            n176 = local read "Time(sec)"() -> (w224:dbl)
            n177 = local read "FreeRun"() -> (w211:bool)
            n178 = local read "Window"() -> (w225:u16)
            n179 = local read "n points"() -> (w219:i32)
            n180 = local read "Lin/Exp"() -> (w220:i32)
            n181 = local read "Correct"() -> (w217:bool)
            n182 = local read "A/M/M"() -> (w216:i32)
            n183 = local read "Mode"() -> (w222:u32)
            n184 = local read "Slope"() -> (w215:u32)
            n185 = global read "CRYMisc vis settings global.vi" "Scope-FFT settings"() -> (w203:T12)
            n186 = Bundle By Name(cluster=w203, "window"=w225, "n avgs"=w221, "lin/exp avg"=w220, "pwr/cplx avg"=w223, "time (ms)"=w224, "fft lines"=w219, "scope/fft mode"=w222, "channel"=w206, "trig. channel"=w218, "Applay Correction"=w217, "Time Display"="", "Freq. Weighting"=w204, "Ave/Max/Min"=w216, "Trigger Level"=w212, "Trigger Unit"=w214, "Trigger Time Offset"=w213, "Trigger Slope"=w215, "Trigger/Free Run"=w211, "continuous"=FALSE, "Spectrum Display"="", "Calc FFT"=w210, "Y-axis"=w202, "Signal Type"=w205) -> (w201:T12)
            n187 = call "CRYFlatten Scope-FFT.vi"("Scope-FFT settings"=w201) -> ("Flat Scope-FFT settings"=w200:string)  [unwired: 10 out]
            n188 = local write "Configure Data"(w200) -> ()
          }
          frame #1 {
            n189 = local write "Set Configure"(TRUE ("Set Configure")) -> ()
          }
        }
      }
      event "Time graph": Value Change; "Time graph": Autoscale Range Change; "Time graph": Plot Attribute Change; "Time graph": Scale Range Change {
        n190 = event-data() -> ()  [unwired: 5 out]
        n191 = control-ref of="Time graph"() -> (w228:refnum<vi>)
        n192 = call "CRYPaint WaterMark.vi"("Type"="Small", "Graph Ref"=w228) -> ()  [unwired: 10 in]
      }
    }
    n193 = global read "CRYMainGlobal.vi" "Acq Stop"() -> (w187:bool)
    n194 = global read "CRYProject Run Control Global.vi" "Cont Seq"() -> (w186:bool)
    n195 = global read "CRYProject Run Control Global.vi" "Cont Seq"() -> (w185:bool)
    n196 = global read "CRYMainGlobal.vi" "STOP"() -> (w190:bool)
    n197 = local read "cont loop"() -> (w189:bool)
    n198 = local read "Cancel"() -> (w192:bool)
    n199 = Not(x=w189) -> (.not. x?=w188:bool)
    n200 = Compound Arithmetic op=OR(w188, w192, w193, w190, w187, w186, w185) -> (w191:bool)
  }
  n201 = while {
    shift-right: [w253] -> w4
    shift-left: _ -> [w267]
    shift-right: [w265] -> _
    shift-left: _ -> [w262]
    shift-right: [w241] -> _
    shift-left: w2 -> [w286]
    shift-right: [w264] -> w1
    shift-left: _ -> [w261]
    shift-right: [w263] -> _
    shift-left: _ -> [w260]
    tunnel: w3 -> [w274]
    shift-right: [w259] -> _
    shift-left: 0 -> [w236]
    shift-right: [w232] -> _
    shift-left: _ -> [w231]
    i -> [w275]
    stop <- w258 continue-if-true
    # "10"
    # "controls prev vals"
    n202 = global read "CRYMainGlobal.vi" "Acq Stop"() -> (w239:bool)
    n203 = global read "CRYMainGlobal.vi" "STOP"() -> (w240:bool)
    n204 = Or(x=w239, y=w240) -> (x .or. y?=w238:bool)
    n205 = global read "CRYProject Run Control Global.vi" "Cont Seq"() -> (w277:bool)
    n206 = global read "CRYProject Run Control Global.vi" "Aborted"() -> (w246:bool)
    n207 = Array Size(array=w260) -> (size(s)=w278:i32)
    n208 = Bundle("Weighting"="Weighting", "Signal Path"="Signal Path", "Y-axis"="Y-axis", "Time(sec)"="Time(sec)", "Mode"="Mode", "Power/Complex"="Power/Complex", "Harmonic"="Harmonic", "Trigger Level"="Trigger Level", "n points"="n points", "Lin/Exp"="Lin/Exp", "Trigger Offset(sec)"="Trigger Offset(sec)", "Trigger Unit"="Trigger Unit", "Averages"="Averages", "Start"="Start", "Spectral Lines"="Spectral Lines", "A/M/M"="A/M/M", "FreeRun"="FreeRun") -> (w287:T10)  [unwired: 1 out]
    n209 = Or(x="OK", y=w277) -> (x .or. y?=w276:bool)
    n210 = Or(x="Cancel", y=w246) -> (x .or. y?=w250:bool)
    n211 = Equal To 0?(x=w275) -> (x = 0?=w268:bool)
    n212 = while {
      shift-right: [w778] -> w269
      shift-left: w267 -> [w779]
      tunnel: "Signal Path" -> [w744]
      tunnel: w262 -> [w780]
      tunnel: "Y-axis" -> [w775]
      tunnel: "Save" -> [w776]
      tunnel: w268 -> [w777]
      tunnel: w250 -> [w773]
      tunnel: w246 -> [w772]
      tunnel: "Continue" -> [w771]
      shift-right: [w769] -> w241
      shift-left: w287 -> [w770]
      tunnel: w286 -> [w768]
      tunnel: "Time(sec)" -> [w741]
      tunnel: "Mode" -> [w767]
      tunnel: "Power/Complex" -> [w766]
      tunnel: "Harmonic" -> [w765]
      tunnel: "Trigger Level" -> [w764]
      tunnel: "Trigger Offset(sec)" -> [w763]
      tunnel: w261 -> [w762]
      tunnel: w278 -> [w761]
      tunnel: w277 -> [w760]
      tunnel: w276 -> [w757]
      tunnel: w275 -> [w756]
      tunnel: "Start" -> [w750]
      tunnel: w274 -> [w755]
      tunnel: "Averages" -> [w754]
      tunnel: "Lin/Exp" -> [w753]
      tunnel: "n points" -> [w752]
      tunnel: "Trigger Unit" -> [w751]
      tunnel: w238 -> [w749]
      tunnel: "CalSpectrum" -> [w748]
      tunnel: "Spectral Lines" -> [w747]
      tunnel: "A/M/M" -> [w746]
      tunnel: "Weighting" -> [w745]
      tunnel: "FreeRun" -> [w743]
      tunnel: w231 -> [w742]
      i -> [w774]
      stop <- w758 continue-if-true
      n213 = case shown="10" w774 {
        tunnel: w779 -> [w785 w797 w926 w982 w1014 w1028 w1111 w1131 w1163 w1215 w1268 w1367 w1408 w1428 w1457 w1477 w1530 w1553 w1599 w1619 w1644]
        tunnel: [w784 w798 w925 w981 w1013 w1027 w1111 w1130 w1162 w1214 w1267 w1366 w1407 w1427 w1456 w1476 w1529 w1552 w1606 w1618 w1635] -> w778
        tunnel: w744 -> [_ _ _ _ _ _ _ _ _ _ w1261 _ _ _ _ _ _ _ _ _ _]
        tunnel: w780 -> [_ _ _ _ _ _ _ _ _ _ _ _ _ _ _ w1472 _ _ _ _ w1641]
        tunnel: w775 -> [_ w796 _ _ _ _ _ _ _ _ _ _ w1403 _ _ w1473 _ _ _ _ w1645]
        tunnel: w776 -> [_ w789 _ _ _ _ _ _ _ _ _ _ _ _ _ _ _ _ _ _ _]
        tunnel: w777 -> [w783 _ w922 w985 _ _ _ w1124 w1159 _ w1265 w1364 w1400 w1426 w1459 w1481 w1531 _ _ _ _]
        tunnel: [FALSE FALSE w918 w983 w1010 FALSE FALSE w1127 FALSE FALSE w1263 w1363 w1399 w1420 w1454 FALSE FALSE FALSE FALSE FALSE TRUE] -> w759
        tunnel: w773 -> [_ _ _ _ w1012 _ _ _ _ _ _ _ _ _ _ _ _ _ _ _ _]
        tunnel: w772 -> [_ _ _ _ _ _ _ _ _ _ _ _ _ _ _ _ _ _ _ _ _]
        tunnel: w771 -> [_ _ _ _ _ w1029 _ _ _ _ _ _ _ _ _ _ _ _ _ _ _]
        tunnel: w770 -> [w781 w795 w921 w988 w1011 w1031 w1114 w1132 w1156 w1210 w1259 w1362 w1402 w1424 w1455 w1484 w1528 w1545 w1601 w1622 w1646]
        tunnel: [w781 w795 w920 w987 w1011 w1030 w1113 w1132 w1155 w1210 w1259 w1361 w1402 w1425 w1455 w1484 w1527 w1544 w1601 w1622 w1646] -> w769
        tunnel: w768 -> [_ _ w928 w990 _ w1032 w1116 w1125 w1160 w1205 w1260 w1370 w1404 _ w1462 w1482 w1532 w1550 w1604 w1623 _]
        tunnel: w741 -> [_ _ w924 _ _ w1026 _ _ _ _ _ _ _ _ _ _ _ w1547 _ _ _]
        tunnel: w767 -> [_ w793 _ w989 _ _ _ _ _ _ _ w1359 _ _ _ _ _ _ _ _ w1640]
        tunnel: w766 -> [_ _ _ _ _ _ _ _ _ _ _ _ _ _ w1460 _ _ _ _ _ _]
        tunnel: w765 -> [_ _ _ _ _ _ _ _ _ _ _ _ _ _ _ w1467 _ _ _ _ _]
        tunnel: w764 -> [_ _ _ _ _ _ _ _ _ _ _ _ _ _ _ _ w1526 _ _ _ _]
        tunnel: w763 -> [_ _ _ _ _ _ _ _ _ _ _ _ _ _ _ _ _ w1546 _ _ _]
        tunnel: w762 -> [_ w794 _ _ _ _ _ _ _ _ _ _ _ _ _ w1471 _ _ w1597 _ _]
        tunnel: w761 -> [_ _ _ _ _ _ _ _ _ _ _ _ _ _ _ w1468 _ _ _ _ _]
        tunnel: w760 -> [_ _ _ _ _ _ _ _ _ _ _ _ _ _ _ _ _ _ _ _ _]
        tunnel: w757 -> [_ w791 _ _ _ _ _ _ _ _ _ _ _ _ _ _ _ _ _ _ _]
        tunnel: w756 -> [_ _ _ _ _ w1035 _ _ _ _ _ w1358 _ _ _ _ _ _ _ _ _]
        tunnel: w755 -> [_ _ _ _ _ _ _ _ _ w1209 _ _ _ _ _ _ _ _ _ _ _]
        tunnel: w754 -> [_ _ _ _ _ w1036 w1112 _ _ w1208 _ _ _ _ _ _ _ _ _ _ _]
        tunnel: w753 -> [_ _ _ _ _ w1025 _ w1126 _ w1206 _ _ _ _ _ _ _ _ _ _ _]
        tunnel: w752 -> [_ _ _ _ _ _ _ _ _ _ _ _ _ w1421 _ _ _ _ _ _ _]
        tunnel: w751 -> [_ _ _ _ _ _ _ _ _ _ _ _ _ _ _ _ _ _ w1596 _ _]
        tunnel: w750 -> [_ _ _ _ _ w1024 _ w1123 w1153 w1204 _ _ _ _ _ _ _ _ _ _ _]
        tunnel: w749 -> [_ _ _ _ w1009 _ _ _ _ _ _ _ _ _ _ _ _ _ _ _ _]
        tunnel: w748 -> [_ _ _ _ _ _ _ _ _ _ _ _ _ _ _ _ _ _ _ _ w1642]
        tunnel: w747 -> [_ _ _ _ _ _ _ _ _ _ _ w1360 _ _ _ _ _ _ _ _ _]
        tunnel: w746 -> [_ _ _ _ _ _ _ _ _ _ _ _ _ _ _ _ _ _ _ _ _]
        tunnel: w745 -> [_ _ _ _ _ _ _ _ w1157 _ _ _ _ _ _ _ _ _ _ _ _]
        tunnel: w743 -> [_ _ _ _ _ _ _ _ _ _ _ _ _ _ _ _ _ _ _ w1620 _]
        tunnel: w742 -> [_ w788 _ _ _ _ _ _ _ _ _ _ _ _ _ _ _ _ _ _ _]
        frame 0 {
          # "initialize"
          n214 = case shown="True" w783 {
            tunnel: [w786 T16 {"acquire"=FALSE, "halt acq"=FALSE, "cal factor"=1.0, "n avgd"=0, "db-pr factor"=1.0, "points"=0, "buffers"=0, "points chg"=TRUE, "db ref"=1.0, "df"=1.0, "window constants"={"eq noise BW"=1.0, "coherent gain"=1.0}, "cursor index"=0, "cursor x"=0.0, "trig level"=0, "est freq"=0.0, "est power"=0.0, "update"=FALSE, "autoscale"=FALSE, "avg. complete"=0, "prebuffer"=0, "nextbuffer"=0, "addbuffs"=0, "Y-axis chg"=FALSE, "Weight"=[]}] -> w784
            tunnel: w785 -> [w786 _]
            frame False {
            }
            frame True {
            }
          }
        }
        frame 1 {
          # "?????????"
          # "Save curve into MemoryList"
          n215 = Or(x=w791, y=w789) -> (x .or. y?=w790:bool)
          n216 = case shown="True" w790 {
            tunnel: [w799 w806] -> w798
            tunnel: w797 -> [w799 w803]
            tunnel: w796 -> [_ w804]
            tunnel: w794 -> [_ w809]
            tunnel: w793 -> [_ w808]
            tunnel: w791 -> [_ w807]
            tunnel: w789 -> [_ w801]
            tunnel: w788 -> [_ w800]
            frame False {
            }
            frame True {
              n217 = local read "Manual"() -> (w802:bool)
              n218 = local write "Save"(FALSE ("save")) -> ()
              n219 = case shown="False" w802 {
                tunnel: w809 -> [w815 _]
                tunnel: w808 -> [w814 _]
                tunnel: w804 -> [w813 _]
                tunnel: w803 -> [w812 _]
                tunnel: w801 -> [w811 _]
                tunnel: w800 -> [w810 _]
                frame False {
                  n220 = case shown="True" w811 {
                    tunnel: w815 -> [_ w824]
                    tunnel: w814 -> [_ w817]
                    tunnel: w813 -> [_ w823]
                    tunnel: w812 -> [_ w822]
                    tunnel: w810 -> [_ w816]
                    frame False {
                    }
                    frame True {
                      n221 = property on="Signal Path" class="Ring (strict)"() -> ("RingText.Text"=w818:string)  [unwired: 2 in, 2 out]
                      n222 = Concatenate Strings(" [" ("string"), w818, "]" ("string")) -> (w819:string)
                      n223 = case shown="1" w817 {
                        tunnel: w819 -> [w845 w853]
                        tunnel: w824 -> [w829 w852]
                        tunnel: w823 -> [_ w850]
                        tunnel: w822 -> [_ w851]
                        tunnel: w818 -> [w832 _]
                        tunnel: w816 -> [w825 _]
                        frame 0, Default {
                          w839 = TRUE ("display X")
                          n224 = local read "Calibration All Cluster"() -> (w827:T1)
                          n225 = local read "dT(sec)"() -> (w831:dbl)
                          n226 = Array Size(array=w829) -> (size(s)=w828:i32)
                          n227 = Flatten To String(anything=w827) -> (data string=w837:string)  [unwired: 1 in, 4 out]
                          n228 = Reciprocal(x=w831) -> (1/x=w830:dbl)
                          n229 = local read "Y Unit"() -> (w840:string)
                          n230 = call "CRYUnflatten Test Infor.vi"() -> ("unflattened test infor data"=w836:T17)  [unwired: 1 in, 9 out]
                          n231 = Bundle By Name(cluster=w836, "Stimulus Type"="WAV", "Signal Type"=w832, "In/Out"=TRUE, "Sampling Rate"=w830, "Samples"=w828, "Calibration Param"=w837) -> (w835:T17)
                          n232 = Concatenate Strings("Oscilloscope WaveForm", w845) -> (w841:string)
                          n233 = call "CRYFlatten Test Infor.vi"("Test Infor data"=w835) -> ("Fattened Data"=w833:string)  [unwired: 10 out]
                          n234 = Bundle By Name(cluster="Waveform Cluster", "protected"=TRUE, "Name"=w841, "Waveform.dX"=w831, "Waveform.Y"=w825, "Plot Settings.Color"=u32 16762922, "X unit"="s" ("Bundle Element"), "Y unit"=w840, "display X"=w839, "display Y"=w839, "Test Info"=w833) -> (w838:T5)
                          n235 = Build Array(w838) -> (w843:T5[])
                          n236 = call "CRYInsert Socket.vi"("sOption1"="Protect" ("sOption"), "Waves"=w843) -> ()  [unwired: 9 in, 1 out]
                        }
                        frame 1 {
                          n237 = stacked-sequence {
                            seq-local: [w858 _] -> [_ w893]
                            tunnel: w853 -> [w876 w906]
                            tunnel: w852 -> [w865 _]
                            tunnel: w851 -> [w870 w904]
                            tunnel: w850 -> [w862 w905]
                            frame #0 {
                              w857 = TRUE ("protected")
                              n238 = Unbundle By Name(w870) -> ("df"=w871:dbl, "db ref"=w861:dbl)
                              n239 = local read "Y Unit"() -> (w859:string)
                              n240 = for {
                                tunnel: w871 -> [w888]
                                tunnel: w865 -> [w886] mode=indexing
                                tunnel: [w883] -> w872 mode=indexing
                                i -> [w887]
                                n241 = Multiply(x=w888, y=w887) -> (x*y=w884:dbl)
                                n242 = Bundle(w884, w886, 0.0) -> (w883:cluster{dbl, dbl, dbl})  [unwired: 1 out]
                              }
                              n243 = case shown="0, Default" w862 {
                                tunnel: [w879 w882] -> w858
                                tunnel: w861 -> [w880 _]
                                tunnel: w859 -> [w878 w882]
                                frame 0, Default {
                                n244 = Format Into String(format string="dB re %.p %s", w880, w878) -> (resulting string=w879:string)  [unwired: 2 in, 1 out]
                                }
                                frame 1 {
                                }
                              }
                              n245 = Concatenate Strings("FFT Spectrum", w876) -> (w868:string)
                              n246 = call "CRYUnflatten Data.vi"() -> ("Datum"=w854:T3)  [unwired: 9 in, 2 out]
                              n247 = Bundle By Name(cluster=w854, "Name"=w868, "X unit"="Hz" ("Bundle Element"), "Y unit"=w858, "Curve"=w872, "X data"=u16 1 ("Bundle Element"), "Y data"=w862, "X axis"=u16 0, "Y axis"=u16 1 ("Bundle Element"), "Y dB ref"=w861, "Plot Settings.Color"=u32 2793216, "single val"=FALSE, "protected"=TRUE, "display X"=w857, "display Y"=w857, "display Z"=FALSE ("protected")) -> (w855:T3)
                              n248 = Build Array(w855) -> (w864:T3[])
                              n249 = call "CRYInsert Socket.vi"("sOption1"="Protect" ("sOption"), "Curves"=w864) -> ()  [unwired: 9 in, 1 out]
                            }
                            frame #1 {
                              w892 = TRUE ("single val")
                              w894 = TRUE ("single val")
                              n250 = local read "dB Est.Level"() -> (w899:dbl)
                              n251 = Unbundle By Name(w904) -> ("db ref"=w908:dbl)
                              n252 = local read "Hz"() -> (w900:dbl)
                              n253 = Bundle("Hz"=w900, "dB Est.Level"=w899, 0.0) -> (w909:cluster{"Hz":dbl, "dB Est.Level":dbl, dbl})  [unwired: 1 out]
                              n254 = Build Array(w909) -> (w902:cluster{"Hz":dbl, "dB Est.Level":dbl, dbl}[])
                              n255 = Concatenate Strings("FFT Cursor", w906) -> (w898:string)
                              n256 = call "CRYUnflatten Data.vi"() -> ("Datum"=w889:T3)  [unwired: 9 in, 2 out]
                              n257 = Bundle By Name(cluster=w889, "Name"=w898, "X unit"="Hz" ("Bundle Element"), "Y unit"=w893, "Curve"=w902, "X data"=u16 1 ("Bundle Element"), "Y data"=w905, "X axis"=u16 0, "Y axis"=u16 1 ("Bundle Element"), "Y dB ref"=w908, "Plot Settings.Color"=u32 16762922, "single val"=w894, "protected"=w894, "display X"=w892, "display Y"=w892, "display Z"=FALSE ("single val")) -> (w890:T3)
                              n258 = Build Array(w890) -> (w896:T3[])
                              n259 = call "CRYInsert Socket.vi"("sOption1"="Protect" ("sOption"), "Values"=w896) -> ()  [unwired: 9 in, 1 out]
                            }
                          }
                        }
                      }
                    }
                  }
                }
                frame True {
                }
              }
              n260 = case shown="True" w807 {
                tunnel: w803 -> [w913 w915]
                tunnel: [w913 w914] -> w806
                frame False {
                }
                frame True {
                  w917 = FALSE ("cont loop")
                  # "OK (T)"
                  n261 = local write "cont loop"(w917) -> ()
                  n262 = local write "Continue"(w917) -> ()
                  n263 = local write "Start"(w917) -> ()
                  n264 = property on="Continue" class="Bool (strict)"("Visible"=w917) -> ()  [unwired: 2 in, 2 out]
                  n265 = Bundle By Name(cluster=w915, "halt acq"=TRUE ("Bundle Element")) -> (w914:T16)
                }
              }
            }
          }
        }
        frame 2 {
          # "Record Time Change"
          n266 = Unbundle By Name(w928) -> ("Time(sec)"=w927:dbl)
          n267 = Not Equal?(x=w927, y=w924) -> (x != y?=w923:bool)
          n268 = Compound Arithmetic op=AND(w923, invert w922) -> (w918:bool)
          n269 = Compound Arithmetic op=OR(w922, w923) -> (w919:bool)
          n270 = case shown="True" w919 {
            tunnel: [w930 w960] -> w925
            tunnel: w926 -> [w930 w961]
            tunnel: w924 -> [_ w931]
            tunnel: w921 -> [w929 w958]
            tunnel: [w929 w959] -> w920
            frame False {
            }
            frame True {
              w943 = 20.0 ("buffer/ms")
              n271 = local read "Sampling rate"() -> (w941:u32)
              n272 = local read "Trigger Offset(sec)"() -> (w949:dbl)
              n273 = disable-structure shown="Disabled" {
                disable-tunnel: w958 -> [w966 _]
                disable-tunnel: w931 -> [w965 _]
                frame Disabled {
                  n274 = property on="Time graph" class="WFGraph (strict)"() -> ("XScale.ScaleFit"=w964:u8)  [unwired: 2 in, 2 out]
                  n275 = case shown="2" w964 {
                    tunnel: w966 -> [_ w969]
                    tunnel: w965 -> [_ w967]
                    frame 0, Default {
                    }
                    frame 2 {
                      n276 = Unbundle By Name(w969) -> ("Mode"=w968:u32)
                      n277 = case shown="0, Default" w968 {
                        tunnel: w967 -> [w970 _]
                        frame 0, Default {
                          n278 = property on="Time graph" class="WFGraph (strict)"("XScale.Minimum"=0.0 ("X Scale.Range:Minimum"), "XScale.Maximum"=w970) -> ()  [unwired: 2 in, 2 out]
                        }
                        frame 1 {
                          n279 = local read "Sampling rate"() -> (w974:u32)
                          n280 = Divide(x=w974, y=2.0) -> (x/y=w972:dbl)
                          n281 = property on="Spectrum graph" class="WFGraph (strict)"("XScale.Minimum"=0.0 ("X Scale.Range:Minimum"), "XScale.Maximum"=w972) -> ()  [unwired: 2 in, 2 out]
                        }
                      }
                    }
                  }
                }
                frame Enabled {
                }
              }
              n282 = Multiply(x=0.05, y=w941) -> (x*y=w944:dbl)
              n283 = Divide(x=w941, y=2.0) -> (x/y=w955:dbl)
              n284 = Reciprocal(x=w931) -> (1/x=w957:dbl)
              n285 = Multiply(x=w931, y=w943) -> (x*y=w963:dbl)
              n286 = local write "dF(Hz)"(w957) -> ()
              n287 = Multiply(x=w943, y=w949) -> (x*y=w945:dbl)
              n288 = To Long Integer(number=w963) -> (32bit integer=w936:i32)
              n289 = Multiply(x=w936, y=w944) -> (x*y=w934:dbl)
              n290 = Multiply(x=w931, y=w955) -> (x*y=w954:dbl)
              n291 = Absolute Value(x=w945) -> (abs(x)=w947:dbl)
              n292 = Negate(x=w931) -> (-x=w932:dbl)
              n293 = Round Toward -Infinity(1:w954) -> (0:w951:dbl)
              n294 = Round Toward +Infinity(x=w947) -> (ceil(x): smallest int >= x=w946:dbl)
              n295 = Less Than 0?(x=w945) -> (x < 0?=w948:bool)
              n296 = Logarithm Base 2(1:w934) -> (0:w953:dbl)
              n297 = property on="Trigger Offset(sec)" class="DigNum (strict)"("Maximum"=w931) -> ()  [unwired: 2 in, 2 out]
              n298 = property on="Trigger Offset(sec)" class="DigNum (strict)"("Minimum"=w932) -> ()  [unwired: 2 in, 2 out]
              n299 = case shown="True" w948 {
                tunnel: w946 -> [_ w980]
                tunnel: [0 w979] -> w940
                tunnel: [2 1] -> w938
                tunnel: w944 -> [_ _]
                frame False {
                }
                frame True {
                  n300 = To Long Integer(number=w980) -> (32bit integer=w979:i32)
                }
              }
              n301 = Round Toward -Infinity(1:w953) -> (0:w952:dbl)
              n302 = Power Of 2(x=w952) -> (2^x=w950:dbl)
              n303 = To Long Integer(number=w950) -> (32bit integer=w935:i32)
              n304 = local read "FreeRun"() -> (w933:bool)
              n305 = local write "Spectral Lines"(w951) -> ()
              n306 = Bundle By Name(cluster=w958, "n points"=w935, "Spectral Lines"=w951, "Time(sec)"=w931) -> (w959:T10)
              n307 = Select(t=0, s=w933, f=w938) -> (s? t:f=w937:i32)
              n308 = local write "n points"(w935) -> ()
              n309 = Bundle By Name(cluster=w961, "points chg"=TRUE ("Bundle Element"), "points"=w935, "prebuffer"=w940, "buffers"=w936, "nextbuffer"=w938, "addbuffs"=w937) -> (w960:T16)
            }
          }
        }
        frame 3 {
          # "scope mode change"
          n310 = Unbundle By Name(w990) -> ("Mode"=w991:u32)
          n311 = Not Equal?(x=w991, y=w989) -> (x != y?=w984:bool)
          n312 = Compound Arithmetic op=OR(w984, w985) -> (w986:bool)
          n313 = Compound Arithmetic op=AND(w984, invert w985) -> (w983:bool)
          n314 = case shown="True" w986 {
            tunnel: w989 -> [_ w999]
            tunnel: w988 -> [w993 w1000]
            tunnel: [w993 w1001] -> w987
            tunnel: w982 -> [w992 w998]
            tunnel: [w992 w996] -> w981
            frame False {
            }
            frame True {
              w994 = u8 2 ("Write Attribute")
              n315 = Equal To 0?(x=w999) -> (x = 0?=w995:bool)
              n316 = Not(x=w995) -> (.not. x?=w1004:bool)
              n317 = Select(t=u8 2 ("Write Attribute"), s=w995, f=u8 0 ("Write Attribute")) -> (s? t:f=w1005:u8)
              n318 = Select(t=w994, s=w995, f=u8 1 ("Write Attribute")) -> (s? t:f=w1002:u8)
              n319 = property on="Window" class="Ring (strict)"("禁用"=w1005) -> ()  [unwired: 2 in, 2 out]
              n320 = property on="Weighting" class="Ring (strict)"("禁用"=w1005) -> ()  [unwired: 2 in, 2 out]
              n321 = property on="Spectral Lines" class="DigNum (strict)"("禁用"=w1005) -> ()  [unwired: 2 in, 2 out]
              n322 = property on="A/M/M" class="Slide (strict)"("禁用"=w1005) -> ()  [unwired: 2 in, 2 out]
              n323 = property on="Power/Complex" class="Slide (strict)"("禁用"=w1005) -> ()  [unwired: 2 in, 2 out]
              n324 = property on="Correct" class="Bool (strict)"("禁用"=w994) -> ()  [unwired: 2 in, 2 out]
              n325 = property on="dF(Hz)" class="DigNum (strict)"("禁用"=w1002) -> ()  [unwired: 2 in, 2 out]
              n326 = property on="Y-axis" class="Ring (strict)"("Visible"=w1004) -> ()  [unwired: 2 in, 2 out]
              n327 = property on="Scale" class="Bool (strict)"("Visible"=w1004) -> ()  [unwired: 2 in, 2 out]
              n328 = property on="Spectrum graph" class="WFGraph (strict)"("Visible"=w1004) -> ()  [unwired: 2 in, 2 out]
              n329 = property on="CalSpectrum" class="Bool (strict)"("Visible"=w995) -> ()  [unwired: 2 in, 2 out]
              n330 = property on="Time graph" class="WFGraph (strict)"("Visible"=w995) -> ()  [unwired: 2 in, 2 out]
              n331 = case shown="False" w995 {
                frame False {
                  n332 = property on="CalSpectrum" class="Bool (strict)"("Value"=TRUE ("CalSpectrum")) -> ()  [unwired: 2 in, 2 out]
                }
                frame True {
                }
              }
              n333 = Bundle By Name(cluster=w1000, "Mode"=w999) -> (w1001:T10)
              n334 = Bundle By Name(cluster=w998, "Y-axis chg"=TRUE) -> (w996:T16)
            }
          }
        }
        frame 4 {
          # "Cancel or stop"
          n335 = Compound Arithmetic op=OR(w1012, w1009) -> (w1010:bool)
          n336 = case shown="True" w1010 {
            tunnel: w1014 -> [w1015 w1018]
            tunnel: [w1015 w1017] -> w1013
            frame False {
            }
            frame True {
              w1016 = FALSE ("Start")
              n337 = Bundle By Name(cluster=w1018, "halt acq"=TRUE ("Bundle Element")) -> (w1017:T16)
              n338 = local write "cont loop"(w1016) -> ()
              n339 = local write "Continue"(w1016) -> ()
              n340 = local write "Cancel"(w1016) -> ()
              n341 = local write "Start"(w1016) -> ()
              n342 = property on="Continue" class="Bool (strict)"("Visible"=w1016) -> ()  [unwired: 2 in, 2 out]
            }
          }
        }
        frame 5 {
          # "???"
          # "first, auto start"
          # "start(continue)"
          n343 = Unbundle By Name(w1032) -> ("Start"=w1023:bool)
          n344 = Equal?(x=w1035, y=1) -> ()  [unwired: 1 out]
          n345 = Not Equal?(x=w1023, y=w1024) -> (x != y?=w1022:bool)
          n346 = And(x=w1022, y=w1024) -> (x .and. y?=w1033:bool)
          n347 = Compound Arithmetic op=OR(w1033, w1029) -> (w1021:bool)
          n348 = case shown="True" w1021 {
            tunnel: w1028 -> [w1039 w1064]
            tunnel: [w1038 w1065] -> w1027
            tunnel: w1036 -> [_ w1079]
            tunnel: w1031 -> [w1041 w1080]
            tunnel: [w1040 w1077] -> w1030
            tunnel: w1029 -> [_ w1073]
            tunnel: w1026 -> [_ w1076]
            tunnel: w1025 -> [w1037 w1074]
            tunnel: w1024 -> [_ _]
            tunnel: w1022 -> [w1042 _]
            frame False {
              # "Stop"
              n349 = case shown="True" w1042 {
                tunnel: w1041 -> [w1044 w1056]
                tunnel: [w1044 w1055] -> w1040
                tunnel: w1039 -> [w1043 w1054]
                tunnel: [w1043 w1053] -> w1038
                tunnel: w1037 -> [_ w1049]
                frame False {
                }
                frame True {
                  w1045 = 0.0 ("timeOut")
                  w1046 = u8 0 ("nSampleFreq")
                  w1058 = u32 0 ("nSampleFreq")
                  n350 = Equal To 0?(x=w1049) -> (x = 0?=w1048:bool)
                  n351 = property on="Continue" class="Bool (strict)"("Visible"=w1048) -> ()  [unwired: 2 in, 2 out]
                  n352 = local read "Device In"() -> (w1060:u32)
                  n353 = local read "taskID"() -> (w1061:u32)
                  n354 = Bundle By Name(cluster=w1056, "Start"=FALSE) -> (w1055:T10)
                  n355 = Bundle By Name(cluster=w1054, "acquire"=FALSE, "halt acq"=TRUE) -> (w1053:T16)
                  n356 = property on="AvgT" class="Bool (strict)"("Value"=FALSE ("AvgT")) -> ()  [unwired: 2 in, 2 out]
                  n357 = dll-call lib="D:/A_CRYSoundLab_Work/CRY6181/CRYSound.dll" fn="GVContinueRecord"("DeviceID"=w1060, "nSampleFreq"=w1058, "nChannels"=w1058, "BitDepth"=w1058, "TimeRate"=w1045, "mode"=w1058, "nBufferUse"=w1058, "RealTime"=w1058, "timeOut"=w1045, "RecData"=i32[] [], "RecDataLen"=w1058, "OverHead"=w1046, "StartFlag"=w1046, "PauseFlag"=w1046, "ChangeFlag"=w1046, "taskID"=w1061) -> ()  [unwired: 10 in, 12 out]
                  n358 = local write "Start"(FALSE ("Start")) -> ()
                }
              }
            }
            frame True {
              n359 = case shown="0, Default" w1074 {
                frame 0, Default {
                  n360 = property on="Avg. Complete" class="DigNum (strict)"("Visible"=TRUE) -> ()  [unwired: 2 in, 2 out]
                  n361 = property on="AvgT" class="Bool (strict)"("Visible"=FALSE ("AvgT")) -> ()  [unwired: 2 in, 2 out]
                }
                frame 1 {
                  n362 = property on="AvgT" class="Bool (strict)"("Visible"=TRUE ("AvgT")) -> ()  [unwired: 2 in, 2 out]
                  n363 = property on="AvgT" class="Bool (strict)"("Value"=TRUE ("AvgT")) -> ()  [unwired: 2 in, 2 out]
                }
              }
              n364 = case shown="True" w1073 {
                tunnel: w1064 -> [w1097 w1099]
                tunnel: [w1096 w1100] -> w1066
                tunnel: w1079 -> [_ w1105]
                frame False {
                  w1095 = 0 ("Bundle Element")
                  n365 = Bundle By Name(cluster=w1097, "acquire"=TRUE ("Bundle Element"), "halt acq"=FALSE, "n avgd"=w1095, "avg. complete"=w1095) -> (w1096:T16)
                }
                frame True {
                  n366 = Unbundle By Name(w1099) -> ("n avgd"=w1104:i32)
                  n367 = Bundle By Name(cluster=w1099, "acquire"=TRUE ("Bundle Element"), "halt acq"=FALSE) -> (w1102:T16)
                  n368 = Less Or Equal?(x=w1105, y=w1104) -> (x <= y?=w1103:bool)
                  n369 = case shown="True" w1103 {
                    tunnel: w1102 -> [w1107 w1109]
                    tunnel: [w1107 w1108] -> w1100
                    frame False {
                    }
                    frame True {
                      n370 = Bundle By Name(cluster=w1109, "n avgd"=0) -> (w1108:T16)
                    }
                  }
                }
              }
              n371 = Unbundle By Name(w1064) -> ("nextbuffer"=w1063:i32)
              n372 = Bundle By Name(cluster=w1080, "Start"=TRUE) -> (w1077:T10)
              n373 = property on="Time graph" class="WFGraph (strict)"() -> ("XScale.ScaleFit"=w1078:u8)  [unwired: 2 in, 2 out]
              n374 = local write "Continue"(FALSE ("Continue")) -> ()
              n375 = property on="Continue" class="Bool (strict)"("Visible"=FALSE) -> ()  [unwired: 2 in, 2 out]
              n376 = property on="Start" class="Bool (strict)"("Value"=TRUE ("Visible")) -> ()  [unwired: 2 in, 2 out]
              n377 = case shown="2" w1078 {
                tunnel: w1077 -> [_ w1087]
                tunnel: w1076 -> [_ w1085]
                frame 0, Default {
                }
                frame 2 {
                  n378 = Unbundle By Name(w1087) -> ("Mode"=w1086:u32)
                  n379 = case shown="0, Default" w1086 {
                    tunnel: w1085 -> [w1088 _]
                    frame 0, Default {
                      n380 = property on="Time graph" class="WFGraph (strict)"("XScale.Minimum"=0.0 ("X Scale.Range:Minimum"), "XScale.Maximum"=w1088) -> ()  [unwired: 2 in, 2 out]
                    }
                    frame 1 {
                      n381 = local read "Sampling rate"() -> (w1092:u32)
                      n382 = Divide(x=w1092, y=2.0) -> (x/y=w1090:dbl)
                      n383 = property on="Spectrum graph" class="WFGraph (strict)"("XScale.Minimum"=0.0 ("X Scale.Range:Minimum"), "XScale.Maximum"=w1090) -> ()  [unwired: 2 in, 2 out]
                    }
                  }
                }
              }
              n384 = local read "FreeRun"() -> (w1067:bool)
              n385 = Select(t=0, s=w1067, f=w1063) -> (s? t:f=w1069:i32)
              n386 = local write "start_flg"(u8 1 ("start_flg")) -> ()
              n387 = Bundle By Name(cluster=w1066, "addbuffs"=w1069) -> (w1065:T16)
            }
          }
        }
        frame 6 {
          n388 = Unbundle By Name(w1116) -> ("Averages"=w1117:i32)
          n389 = Not Equal?(x=w1117, y=w1112) -> (x != y?=w1115:bool)
          n390 = case shown="True" w1115 {
            tunnel: w1114 -> [w1119 w1122]
            tunnel: [w1119 w1121] -> w1113
            tunnel: w1112 -> [_ w1120]
            frame False {
            }
            frame True {
              n391 = Bundle By Name(cluster=w1122, "Averages"=w1120) -> (w1121:T10)
            }
          }
        }
        frame 7 {
          # "Linear/Exponential"
          n392 = Unbundle By Name(w1125) -> ("Lin/Exp"=w1133:i32)
          n393 = Not Equal?(x=w1133, y=w1126) -> (x != y?=w1129:bool)
          n394 = Or(x=w1124, y=w1129) -> (x .or. y?=w1128:bool)
          n395 = Compound Arithmetic op=AND(w1129, invert w1124) -> (w1127:bool)
          n396 = case shown="True" w1128 {
            tunnel: w1131 -> [w1134 w1140]
            tunnel: [w1134 w1144] -> w1130
            tunnel: w1126 -> [_ w1141]
            tunnel: w1123 -> [_ w1137]
            frame False {
            }
            frame True {
              n397 = Equal To 0?(x=w1141) -> (x = 0?=w1138:bool)
              n398 = property on="AvgT" class="Bool (strict)"("Value"=w1137) -> ()  [unwired: 2 in, 2 out]
              n399 = Not(x=w1138) -> (.not. x?=w1142:bool)
              n400 = property on="Avg. Complete" class="DigNum (strict)"("Visible"=w1138) -> ()  [unwired: 2 in, 2 out]
              n401 = property on="AvgT" class="Bool (strict)"("Visible"=w1142) -> ()  [unwired: 2 in, 2 out]
              n402 = property on="Continue" class="Bool (strict)"("Visible"=FALSE) -> ()  [unwired: 2 in, 2 out]
              n403 = case shown="True" w1138 {
                tunnel: [w1147 w1150] -> w1136
                frame False {
                  n404 = call "CRYGet Error Message.vi"("Error No"=1, "Kind"="Oscilloscope-FFT Sub") -> ("Unicode Message Sub"=w1147:string[])  [unwired: 4 in, 5 out]
                }
                frame True {
                  n405 = call "CRYGet Error Message.vi"("Error No"=0, "Kind"="Oscilloscope-FFT Sub") -> ("Unicode Message Sub"=w1150:string[])  [unwired: 4 in, 5 out]
                }
              }
              n406 = Bundle By Name(cluster=w1140, "n avgd"=0 ("Bundle Element")) -> (w1144:T16)
              n407 = for {
                tunnel: w1136 -> [w1146] mode=indexing
                tunnel: [w1145] -> w1135 mode=indexing
                n408 = call "CRYConvert Unicode to ASCII.vi"("Unicode"=w1146) -> ("ASCII"=w1145:string)  [unwired: 4 in]
              }
              n409 = property on="Start" class="Bool (strict)"("Strings [4]"=w1135) -> ()  [unwired: 2 in, 2 out]
            }
          }
        }
        frame 8 {
          # "Weighting"
          n410 = Unbundle By Name(w1160) -> ("Weighting"=w1164:u16)
          n411 = Not Equal?(x=w1164, y=w1157) -> (x != y?=w1158:bool)
          n412 = Or(x=w1159, y=w1158) -> (x .or. y?=w1161:bool)
          n413 = Compound Arithmetic op=AND(w1158, invert w1159) -> ()  [unwired: 1 out]
          n414 = case shown="True" w1161 {
            tunnel: w1163 -> [w1166 w1179]
            tunnel: [w1166 w1176] -> w1162
            tunnel: w1157 -> [_ w1174]
            tunnel: w1156 -> [w1165 w1182]
            tunnel: [w1165 w1181] -> w1155
            tunnel: w1153 -> [_ w1180]
            frame False {
            }
            frame True {
              n415 = property on="Weighting" class="Ring (strict)"() -> ("Strings []"=w1175:string[])  [unwired: 2 in, 2 out]
              n416 = case shown="True" w1180 {
                tunnel: [w1198 w1201] -> w1177
                tunnel: w1179 -> [w1195 w1199]
                frame False {
                  n417 = Bundle By Name(cluster=w1195, "acquire"=FALSE, "halt acq"=TRUE ("acquire")) -> (w1198:T16)
                }
                frame True {
                  n418 = Bundle By Name(cluster=w1199, "acquire"=TRUE, "halt acq"=FALSE ("acquire")) -> (w1201:T16)
                }
              }
              n419 = Index Array(array=w1175, index=w1174) -> (element=w1173:string)
              n420 = call "CRYGet Weighting Value.vi"("Weighting Name"=w1173) -> ("Weighting Curve"=w1168:T3)  [unwired: 10 in]
              n421 = Unbundle By Name(w1168) -> ("Curve"=w1169:cluster{"x":dbl, "y":dbl, "z":dbl}[], "Y dB ref"=w1170:dbl, "Y data"=w1171:u16)
              n422 = Sort 1D Array(array=w1169) -> (sorted array=w1172:cluster{"x":dbl, "y":dbl, "z":dbl}[])
              n423 = Bundle By Name(cluster=w1182, "Weighting"=w1174) -> (w1181:T10)
              n424 = for {
                tunnel: w1172 -> [w1190] mode=indexing
                tunnel: [w1189] -> w1167 mode=indexing
                tunnel: w1170 -> [w1187]
                tunnel: w1171 -> [w1188]
                n425 = Unbundle(w1190) -> ("x"=w1184:dbl, "y"=w1186:dbl)  [unwired: 1 out]
                n426 = case shown="0" w1188 {
                  tunnel: w1186 -> [w1191 w1194]
                  tunnel: [w1191 w1193] -> w1185
                  tunnel: w1187 -> [_ w1192]
                  frame 1, Default {
                  }
                  frame 0 {
                    n427 = call "CRYConversion dB-Lin.vi"("dB ref."=w1192, "Log In"=w1194) -> ("Lin Out"=w1193:dbl)  [unwired: 4 in, 3 out]
                  }
                }
                n428 = Logarithm Base 10(1:w1184) -> (0:w1183:dbl)
                n429 = Bundle(w1183, "Lin Out"=w1185) -> (w1189:cluster{dbl, "Lin Out":dbl})  [unwired: 1 out]
              }
              n430 = Bundle By Name(cluster=w1177, "Weight"=w1167, "n avgd"=0) -> (w1176:T16)
            }
          }
        }
        frame 9 {
          # "linear averaging count"
          n431 = Unbundle By Name(w1215) -> ("acquire"=w1203:bool, "n avgd"=w1212:i32, "avg. complete"=w1207:i32)
          n432 = Equal To 0?(x=w1206) -> (x = 0?=w1216:bool)
          n433 = And(x=w1216, y=w1203) -> (x .and. y?=w1213:bool)
          n434 = case shown="True" w1213 {
            tunnel: w1215 -> [w1220 w1246]
            tunnel: [w1221 w1245] -> w1214
            tunnel: w1212 -> [w1219 w1242]
            tunnel: w1209 -> [_ w1244]
            tunnel: w1208 -> [w1218 w1243]
            tunnel: w1207 -> [_ w1241]
            tunnel: w1206 -> [_ w1239]
            tunnel: w1205 -> [_ w1237]
            tunnel: w1204 -> [_ w1234]
            tunnel: w1203 -> [w1217 _]
            frame False {
              # "Exponentional"
              n435 = case shown="True" w1217 {
                tunnel: [w1222 w1227] -> w1221
                tunnel: w1220 -> [w1222 w1226]
                tunnel: w1219 -> [_ w1225]
                tunnel: w1218 -> [_ w1223]
                frame False {
                }
                frame True {
                  n436 = Greater Or Equal?(x=w1225, y=w1223) -> (x >= y?=w1224:bool)
                  n437 = case shown="True" w1224 {
                    tunnel: [w1228 w1229] -> w1227
                    tunnel: w1226 -> [w1228 w1229]
                    frame False {
                    }
                    frame True {
                      n438 = Bundle By Name(cluster=w1229, "n avgd"=0) -> ()  [unwired: 1 out]
                    }
                  }
                }
              }
            }
            frame True {
              # "Linear"
              n439 = Unbundle By Name(w1237) -> ("Start"=w1238:bool)
              n440 = Add(x=w1241, y=w1242) -> (x+y=w1240:i32)
              "Avg. Complete" <- w1240
              n441 = Not(x=w1234) -> (.not. x?=w1236:bool)
              n442 = Not Equal?(x=w1238, y=w1234) -> (x != y?=w1235:bool)
              n443 = Greater Or Equal?(x=w1242, y=w1243) -> (x >= y?=w1232:bool)
              n444 = And(x=w1235, y=w1236) -> (x .and. y?=w1233:bool)
              n445 = Or(x=w1233, y=w1232) -> (x .or. y?=w1231:bool)
              n446 = case shown="True" w1231 {
                tunnel: w1246 -> [w1255 w1258]
                tunnel: [w1254 w1258] -> w1245
                tunnel: w1244 -> [w1253 _]
                tunnel: w1240 -> [w1252 _]
                tunnel: w1239 -> [w1251 _]
                frame True {
                  w1250 = FALSE ("Continue")
                  n447 = Equal To 0?(x=w1251) -> (x = 0?=w1249:bool)
                  n448 = case shown="False" w1253 {
                    frame False {
                      n449 = local write "OK"(TRUE ("ok")) -> ()
                    }
                    frame True {
                    }
                  }
                  n450 = local write "Continue"(w1250) -> ()
                  n451 = local write "Start"(w1250) -> ()
                  n452 = Bundle By Name(cluster=w1255, "n avgd"=0, "avg. complete"=w1252, "halt acq"=TRUE ("Bundle Element"), "acquire"=FALSE) -> (w1254:T16)
                  n453 = property on="Continue" class="Bool (strict)"("Visible"=w1249) -> ()  [unwired: 2 in, 2 out]
                }
                frame False {
                }
              }
            }
          }
        }
        frame 10 {
          # "????????????"
          # "Input Channel Changing"
          n454 = Unbundle By Name(w1260) -> ("Signal Path"=w1262:i32)
          n455 = Not Equal?(x=w1262, y=w1261) -> (x != y?=w1264:bool)
          n456 = Compound Arithmetic op=AND(w1264, invert w1265) -> (w1263:bool)
          n457 = Compound Arithmetic op=OR(w1265, w1264) -> (w1266:bool)
          n458 = case shown="True" w1266 {
            tunnel: w1268 -> [w1269 w1270]
            tunnel: [w1269 w1271] -> w1267
            tunnel: w1261 -> [_ _]
            frame False {
            }
            frame True {
              n459 = stacked-sequence {
                tunnel: [_ w1329 _] -> w1271
                tunnel: w1270 -> [_ w1322 _]
                frame #0 {
                  n460 = local read "Audio Driver"() -> (w1272:u16)
                  n461 = case shown="2" w1272 {
                    frame 2 {
                      n462 = local read "ASIO_Inited"() -> (w1275:bool)
                      n463 = case shown="True" w1275 {
                        frame False {
                        }
                        frame True {
                          n464 = local read "Channel In"() -> (w1276:u16)
                          n465 = local read "Asio OCI"() -> (w1277:u32)
                          n466 = local write "ASIO_Inited"(FALSE ("ASIO_Inited")) -> ()
                          n467 = call "CRYASIO Close Cur Channel & Dev.vi"("Limit"=w1277, "isInput?"=TRUE, "Channel Out"=w1276) -> ()  [unwired: 9 in]
                        }
                      }
                      n468 = local read "Rcv Idx"() -> (w1273:u16)
                      n469 = local read "isMain"() -> (w1274:bool)
                      n470 = call "CRYClear Main Receiver Array.vi"("isMain"=w1274, "Rcv Idx"=w1273) -> ()  [unwired: 10 in]
                    }
                    frame 0, Default {
                      w1281 = u32 0 ("nSampleFreq")
                      n471 = local read "Device In"() -> (w1283:u32)
                      n472 = local read "taskID"() -> (w1284:u32)
                      n473 = dll-call lib="D:/A_CRYSoundLab_Work/CRY6181/CRYSound.dll" fn="GVContinueRecord"("DeviceID"=w1283, "nSampleFreq"=w1281, "nChannels"=w1281, "BitDepth"=w1281, "TimeRate"=w1281, "mode"=w1281, "nBufferUse"=w1281, "RealTime"=w1281, "timeOut"=w1281, "RecData"=i32[] [], "RecDataLen"=w1281, "OverHead"=w1281, "StartFlag"=u8 0, "PauseFlag"=w1281, "ChangeFlag"=w1281, "taskID"=w1284) -> ()  [unwired: 10 in, 12 out]
                    }
                  }
                }
                frame #1 {
                  w1294 = 4194303.0  # 2^22 - 1
                  (unwired) 2147483647.0  # 2^31 - 1
                  n474 = local read "Calibration"() -> (w1289:string)
                  n475 = property on="Signal Path" class="Ring (strict)"() -> ("RingText.Text"=w1291:string)  [unwired: 2 in, 2 out]
                  n476 = local read "Hardware"() -> (w1290:string)
                  n477 = local read "Manual"() -> (w1317:bool)
                  n478 = case shown="False" w1317 {
                    tunnel: [w1335 "Y Unit"] -> w1307
                    tunnel: [w1336 "dB ref."] -> w1327
                    tunnel: [w1338 "Sensitivity"] -> w1316
                    frame False {
                      n479 = property on="Signal Path" class="Ring (strict)"() -> ("RingText.Text"=w1341:string)  [unwired: 2 in, 2 out]
                      n480 = call "CRYGet Current Calibration Info.vi"("Is Input?"=TRUE, "Signal Type Name"=w1341) -> ("Calibration All Cluster"=w1334:T1)  [unwired: 9 out]
                      "Calibration All Cluster" <- w1334
                      n481 = Unbundle By Name(w1334) -> ("Sens Curve.Curve"=w1337:cluster{"x":dbl, "y":dbl, "z":dbl}[], "Sens Curve.Y unit"=w1335:string, "Sens Curve.Y dB ref"=w1336:dbl)
                      n482 = Index Array(array=w1337) -> (element=w1339:cluster{"x":dbl, "y":dbl, "z":dbl})  [unwired: 1 in]
                      n483 = Unbundle By Name(w1339) -> ("y"=w1338:dbl)
                      n484 = local write "Sensitivity"(w1338) -> ()
                      n485 = local write "dB ref."(w1336) -> ()
                    }
                    frame True {
                    }
                  }
                  n486 = call "CRYGet Hardware Info From Signal Type.vi"("Calibration In"=w1289, "Hardware In"=w1290, "Signal Type"=w1291, "In/Out?"=TRUE) -> ("Channel Info Out"=w1292:T13)  [unwired: 5 in, 2 out]
                  n487 = Search/Split String(string=w1307, search string/char (-)="/" ("search char (-)")) -> (substring before match=w1311:string, match + rest of string=w1313:string, offset of match=w1309:i32)  [unwired: 1 out]
                  n488 = Unbundle By Name(w1292) -> ("Device Name"=w1287:string, "ID"=w1323:i32, "Hardware Ch ID"=w1285:u8, "Sampling Rate (Hz)"=w1299:u32, "Bit Depth"=w1298:u32, "Vmax (V)"=w1315:dbl, "Audio Driver"=w1286:u16)
                  n489 = case shown="2" w1286 {
                    tunnel: w1285 -> [_ w1332]
                    frame 0, Default {
                      n490 = local read "Rcv Idx"() -> (w1331:u16)
                      n491 = call "CRYUpdate Receiver Index.vi"("Chn Idx"=-1, "Receiver_Index"=w1331) -> ()  [unwired: 9 in]
                    }
                    frame 2 {
                      n492 = local read "Rcv Idx"() -> (w1333:u16)
                      n493 = call "CRYUpdate Receiver Index.vi"("Chn Idx"=w1332, "Receiver_Index"=w1333) -> ()  [unwired: 9 in]
                    }
                  }
                  n494 = String Subset(string=w1313, offset (0)=1) -> (substring=w1314:string)  [unwired: 1 in]
                  n495 = Greater Or Equal To 0?(x=w1309) -> (x >= 0?=w1310:bool)
                  n496 = Select(t=w1314, s=w1310, f=w1311) -> (s? t:f=w1306:string)
                  n497 = Divide(x=w1315, y=w1316) -> (x/y=w1296:dbl)
                  "Max Level" <- w1296
                  n498 = To Unsigned Long Integer(number=w1323) -> (unsigned 32bit integer=w1288:u32)
                  n499 = local write "Y Unit"(w1306) -> ()
                  n500 = call "CRYUnit Prefix to Multiplier.vi"() -> ("multiplier"=w1328:dbl)  [unwired: 1 in, 4 out]
                  n501 = Divide(x=w1296, y=w1294) -> (x/y=w1295:dbl)
                  n502 = local write "Sampling rate"(w1299) -> ()
                  n503 = local write "Device In"(w1288) -> ()
                  n504 = local write "Channel In"(w1285) -> ()
                  n505 = local write "Bits"(w1298) -> ()
                  n506 = local write "Audio Driver"(w1286) -> ()
                  n507 = Build Array("dB", w1306) -> (w1318:string[])
                  n508 = To Double Precision Float(number=w1299) -> (double precision float=w1300:dbl)
                  n509 = To Long Integer(number=w1298) -> (32bit integer=w1301:i32)
                  n510 = Multiply(x=w1327, y=w1328) -> (x*y=w1324:dbl)
                  n511 = property on="Trigger Unit" class="Slide (strict)"("TextLbls[]"=w1318) -> ()  [unwired: 2 in, 2 out]
                  n512 = Bundle(w1300, "32bit integer"=2, w1301) -> (w1303:cluster{dbl, "32bit integer":i32, i32})  [unwired: 1 in]
                  n513 = property on="Spectral Lines" class="DigNum (strict)"("Minimum"=256.0 ("Data Entry Limits:Minimum")) -> ()  [unwired: 2 in, 2 out]
                  n514 = Reciprocal(x=w1299) -> (1/x=w1320:dbl)
                  n515 = call "CRYGet Initialized WFM Array.vi"("Sound Format"=w1303, "Time(s)"=0.05) -> ("initialized array"=w1297:i32[])  [unwired: 8 in, 5 out]
                  n516 = Bundle By Name(cluster=w1322, "db-pr factor"=w1324, "db ref"=w1327, "cal factor"=w1295, "points chg"=TRUE ("Bundle Element"), "update"=TRUE, "Y-axis chg"=TRUE) -> (w1329:T16)
                  n517 = local write "Device Name"(w1287) -> ()
                  n518 = local write "initialized array"(w1297) -> ()
                  n519 = local write "dT(sec)"(w1320) -> ()
                }
                frame #2 {
                  n520 = local read "ASIO_Inited"() -> (w1345:bool)
                  n521 = local read "Audio Driver"() -> (w1346:u16)
                  n522 = case shown="2" w1346 {
                    tunnel: w1345 -> [w1347 _]
                    frame 2 {
                      n523 = case shown="False" w1347 {
                        frame False {
                          n524 = local read "Device Name"() -> (w1356:string)
                          n525 = local read "Sampling rate"() -> (w1354:u32)
                          n526 = local read "Channel In"() -> (w1355:u16)
                          n527 = local read "Bits"() -> (w1353:u32)
                          n528 = local read "Rcv Idx"() -> (w1349:u16)
                          n529 = call "CRYSet Main Receiver Array.vi"("Rcv Idx"=w1349) -> ("Is Main?"=w1350:bool)  [unwired: 10 in]
                          n530 = call "CRYASIO In & Init & Start.vi"("Bit Depth"=w1353, "Sampling Rate"=w1354, "Channel Index"=w1355, "Device Name"=w1356) -> ("bResult"=w1351:bool, "ASIO Opend Channel Index"=→"Asio OCI":u32)  [unwired: 6 in]
                          n531 = local write "ASIO_Inited"(w1351) -> ()
                          n532 = local write "isMain"(w1350) -> ()
                          n533 = local write "Buf Cnt"(-1 ("Buf Cnt")) -> ()
                        }
                        frame True {
                        }
                      }
                    }
                    frame 0, Default {
                      n534 = local write "start_flg"(u8 1 ("start_flg")) -> ()
                    }
                  }
                }
              }
            }
          }
        }
        frame 11 {
          # "Spectral Line Change"
          n535 = Unbundle By Name(w1370) -> ("Spectral Lines"=w1369:dbl)
          n536 = Not Equal?(x=w1369, y=w1360) -> (x != y?=w1365:bool)
          n537 = Or(x=w1364, y=w1365) -> (x .or. y?=w1368:bool)
          n538 = Compound Arithmetic op=AND(w1365, invert w1364) -> (w1363:bool)
          n539 = case shown="True" w1368 {
            tunnel: [w1372 w1382] -> w1366
            tunnel: w1367 -> [w1372 w1382]
            tunnel: w1362 -> [w1371 w1374]
            tunnel: [w1371 w1373] -> w1361
            tunnel: w1360 -> [_ w1381]
            tunnel: w1359 -> [_ w1380]
            tunnel: w1358 -> [_ w1379]
            frame False {
            }
            frame True {
              n540 = Not Equal To 0?(x=w1380) -> (x != 0?=w1376:bool)
              n541 = Greater?(x=w1379, y=1) -> (0:w1377:bool)
              n542 = And(x=w1377, y=w1376) -> (x .and. y?=w1375:bool)
              n543 = case shown="True" w1375 {
                tunnel: w1381 -> [_ w1398]
                tunnel: w1374 -> [w1383 w1391]
                tunnel: [w1383 w1390] -> w1373
                frame False {
                }
                frame True {
                  w1384 = 0.05 ("y")
                  n544 = local read "Sampling rate"() -> (w1395:u32)
                  n545 = Multiply(x=w1398, y=2.0) -> (x*y=w1396:dbl)
                  n546 = Divide(x=w1396, y=w1395) -> (x/y=w1394:dbl)
                  n547 = Quotient & Remainder(x=w1394, y=w1384) -> (x-y*floor(x/y)=w1388:dbl, floor(x/y)=w1386:dbl)
                  n548 = Round Toward +Infinity(x=w1388) -> (ceil(x): smallest int >= x=w1387:dbl)
                  n549 = Add(x=w1387, y=w1386) -> (x+y=w1385:dbl)
                  n550 = Multiply(x=w1385, y=w1384) -> (x*y=w1392:dbl)
                  n551 = Greater?(x=w1392, y=w1384) -> (0:w1393:bool)
                  n552 = Select(t=w1392, s=w1393, f=w1384) -> (s? t:f=w1389:dbl)
                  n553 = local write "Time(sec)"(w1389) -> ()
                  n554 = Bundle By Name(cluster=w1391, "Time(sec)"=w1389) -> (w1390:T10)
                }
              }
            }
          }
        }
        frame 12 {
          # "Y axis Scale Changing"
          n555 = Unbundle By Name(w1404) -> ("Y-axis"=w1405:u16)
          n556 = Not Equal?(x=w1405, y=w1403) -> (x != y?=w1401:bool)
          n557 = Or(x=w1400, y=w1401) -> (x .or. y?=w1406:bool)
          n558 = Compound Arithmetic op=AND(w1401, invert w1400) -> (w1399:bool)
          n559 = case shown="True" w1406 {
            tunnel: w1408 -> [w1409 w1419]
            tunnel: [w1409 w1418] -> w1407
            tunnel: w1403 -> [_ w1417]
            tunnel: w1400 -> [_ w1416]
            frame False {
            }
            frame True {
              n560 = Equal To 0?(x=w1417) -> (x = 0?=w1414:bool)
              n561 = local read "Y Unit"() -> (w1411:string)
              n562 = Not(x=w1416) -> (.not. x?=w1415:bool)
              n563 = Select(t="dB" ("Caption.Text"), s=w1414, f=w1411) -> (s? t:f=w1410:string)
              n564 = Bundle By Name(cluster=w1419, "Y-axis chg"=TRUE, "autoscale"=w1415) -> (w1418:T16)
              n565 = property on="Est.Unit" class="Str"("Text.Text"=w1410) -> ()  [unwired: 2 in, 2 out]
            }
          }
        }
        frame 13 {
          # "n Points Change"
          n566 = Unbundle By Name(w1424) -> ("n points"=w1423:i32)
          n567 = Not Equal?(x=w1423, y=w1421) -> (x != y?=w1422:bool)
          n568 = Compound Arithmetic op=AND(invert w1426, w1422) -> (w1420:bool)
          n569 = case shown="True" w1420 {
            tunnel: w1428 -> [w1430 w1442]
            tunnel: [w1430 w1441] -> w1427
            tunnel: w1424 -> [w1429 w1438]
            tunnel: [w1429 w1437] -> w1425
            tunnel: w1421 -> [_ w1435]
            frame False {
            }
            frame True {
              n570 = local read "Sampling rate"() -> (w1432:u32)
              n571 = Multiply(x=w1432, y=0.05) -> (x*y=w1433:dbl)
              n572 = To Long Integer(number=w1433) -> (32bit integer=w1431:i32)
              n573 = Quotient & Remainder(x=w1435, y=w1431) -> (x-y*floor(x/y)=w1440:i32, floor(x/y)=w1443:i32)
              n574 = Equal To 0?(x=w1440) -> (x = 0?=w1444:bool)
              n575 = case shown="False" w1444 {
                tunnel: [w1451 w1453] -> w1436
                tunnel: w1443 -> [w1452 w1453]
                frame False {
                  n576 = Increment(x=w1452) -> (x+1=w1451:i32)
                }
                frame True {
                }
              }
              n577 = disable-structure shown="Disabled" {
                disable-tunnel: w1438 -> [w1448 w1450]
                disable-tunnel: [w1447 w1450] -> w1437
                disable-tunnel: w1436 -> [w1445 _]
                frame Disabled {
                  # "??????????"
                  n578 = Multiply(x=w1445, y=50.0) -> (x*y=w1446:dbl)
                  n579 = Bundle By Name(cluster=w1448, "Time(sec)"=w1446) -> (w1447:T10)
                  n580 = local write "Time(sec)"(w1446) -> ()
                }
                frame Enabled {
                }
              }
              n581 = Bundle By Name(cluster=w1442, "points chg"=TRUE ("Bundle Element"), "buffers"=w1436, "points"=w1435) -> (w1441:T16)
            }
          }
        }
        frame 14 {
          # "power or complex averaging"
          n582 = Unbundle By Name(w1462) -> ("Power/Complex"=w1461:i32)
          n583 = Not Equal?(x=w1461, y=w1460) -> (x != y?=w1458:bool)
          n584 = Compound Arithmetic op=AND(invert w1459, w1458) -> (w1454:bool)
          n585 = case shown="True" w1454 {
            tunnel: w1457 -> [w1463 w1466]
            tunnel: [w1463 w1465] -> w1456
            frame False {
            }
            frame True {
              n586 = Bundle By Name(cluster=w1466, "points chg"=TRUE) -> (w1465:T16)
            }
          }
        }
        frame 15 {
          # "?????????"
          # "harmonic cursor"
          n587 = Unbundle By Name(w1482) -> ("Harmonic"=w1470:bool, "Y-axis"=w1469:u16)
          n588 = Not Equal?(x=w1469, y=w1473) -> (x != y?=w1479:bool)
          n589 = Exclusive Or(1:w1467, 2:w1470) -> (0:w1480:bool)
          n590 = case shown="True" w1480 {
            tunnel: w1477 -> [w1486 w1497]
            tunnel: [w1486 w1496] -> w1476
            tunnel: [w1485 w1494] -> w1475
            tunnel: [w1485 w1495] -> w1474
            tunnel: w1467 -> [_ w1493]
            frame False {
              w1485 = FALSE
            }
            frame True {
              n591 = property on="Spectrum graph" class="WFGraph (strict)"("活动游标"=u32 0 ("Write Attribute")) -> ("游标.游标锁定样式"=w1487:u32)  [unwired: 2 in, 2 out]
              n592 = Equal To 0?(x=w1487) -> (x = 0?=w1494:bool)
              n593 = case shown="True" w1494 {
                tunnel: w1497 -> [w1500 w1505]
                tunnel: [w1501 w1506] -> w1492
                tunnel: [w1499 w1504] -> w1496
                frame False {
                  n594 = property on="Spectrum graph" class="WFGraph (strict)"() -> ("游标.游标索引"=w1498:i32)  [unwired: 2 in, 2 out]
                  n595 = Unbundle By Name(w1500) -> ("cursor index"=w1502:i32)
                  n596 = Bundle By Name(cluster=w1500, "cursor index"=w1498) -> (w1499:T16)
                  n597 = Not Equal?(x=w1498, y=w1502) -> (x != y?=w1501:bool)
                }
                frame True {
                  n598 = property on="Spectrum graph" class="WFGraph (strict)"() -> ("游标.游标位置:游标X坐标"=w1503:dbl)  [unwired: 2 in, 2 out]
                  n599 = Unbundle By Name(w1505) -> ("cursor x"=w1507:dbl)
                  n600 = Bundle By Name(cluster=w1505, "cursor x"=w1503) -> (w1504:T16)
                  n601 = Not Equal?(x=w1503, y=w1507) -> (x != y?=w1506:bool)
                }
              }
              n602 = Select(t=u8 0 ("Write Attribute"), s=w1493, f=u8 2 ("Write Attribute")) -> (s? t:f=w1489:u8)
              n603 = property on="THD" class="DigNum (strict)"("禁用"=w1489) -> ()  [unwired: 2 in, 2 out]
              n604 = Or(x=w1494, y=w1492) -> (x .or. y?=w1495:bool)
            }
          }
          n605 = Compound Arithmetic op=OR(w1481, w1467, w1474, w1479) -> (w1478:bool)
          n606 = case shown="True" w1478 {
            tunnel: w1476 -> [_ w1523]
            tunnel: w1475 -> [_ w1516]
            tunnel: w1473 -> [_ w1522]
            tunnel: w1472 -> [_ w1521]
            tunnel: w1471 -> [_ w1520]
            tunnel: w1467 -> [_ w1518]
            tunnel: w1468 -> [_ w1517]
            frame False {
            }
            frame True {
              n607 = Equal To 0?(x=w1522) -> (x = 0?=w1519:bool)
              n608 = property on="Spectrum graph" class="WFGraph (strict)"() -> ("原游标列表"=w1509:T18)  [unwired: 2 in, 2 out]
              n609 = Unbundle By Name(w1523) -> ("window constants"=w1511:cluster{"eq noise BW":dbl, "coherent gain":dbl}, "df"=w1512:dbl, "est freq"=w1513:dbl, "est power"=w1514:dbl, "db-pr factor"=w1515:dbl)
              n610 = call "CRYHarmonic cursors4.vi"("Cursor List in"=w1509, "Log data"=w1519, "dB ref"=w1515, "Harm. cursor on"=w1518, "window constants"=w1511, "Estimated power"=w1514, "df"=w1512, "n f points"=w1517, "Cursor free"=w1516, "Power spectrum"=w1521, "Spectrum y"=w1520, "Estimated freq."=w1513) -> ("Cursor List out"=w1508:T19, "THD (%)"=→"THD":dbl)  [unwired: 2 out]
              n611 = property on="Spectrum graph" class="WFGraph (strict)"("原游标列表"=w1508) -> ()  [unwired: 2 in, 2 out]
            }
          }
        }
        frame 16 {
          # "???????????"
          # "trigger (V)"
          n612 = Unbundle By Name(w1532) -> ("Trigger Level"=w1533:dbl)
          n613 = Not Equal?(x=w1533, y=w1526) -> (x != y?=w1534:bool)
          n614 = Or(x=w1531, y=w1534) -> (x .or. y?=w1525:bool)
          n615 = case shown="True" w1525 {
            tunnel: w1530 -> [w1536 w1538]
            tunnel: [w1536 w1539] -> w1529
            tunnel: w1528 -> [w1535 w1541]
            tunnel: [w1535 w1540] -> w1527
            tunnel: w1526 -> [_ w1537]
            frame False {
            }
            frame True {
              n616 = Unbundle By Name(w1538) -> ("cal factor"=w1542:dbl)
              n617 = Divide(x=w1537, y=w1542) -> (x/y=w1543:dbl)
              n618 = Bundle By Name(cluster=w1541, "Trigger Level"=w1537) -> (w1540:T10)
              n619 = Bundle By Name(cluster=w1538, "trig level"=w1543) -> (w1539:T16)
            }
          }
        }
        frame 17 {
          # "??????????????"
          # "trigger offset(second)"
          n620 = Unbundle By Name(w1550) -> ("Trigger Offset(sec)"=w1548:dbl)
          n621 = Not Equal?(x=w1548, y=w1546) -> (x != y?=w1549:bool)
          n622 = case shown="True" w1549 {
            tunnel: w1553 -> [w1555 w1572]
            tunnel: [w1555 w1571] -> w1552
            tunnel: w1547 -> [_ _]
            tunnel: w1546 -> [_ w1568]
            tunnel: w1545 -> [w1554 w1569]
            tunnel: [w1554 w1559] -> w1544
            frame False {
            }
            frame True {
              n623 = local read "Time(sec)"() -> (w1557:dbl)
              n624 = local read "Sampling rate"() -> (w1574:u32)
              n625 = local read "Time(sec)"() -> (w1558:dbl)
              n626 = Less?(x=w1557, y=w1568) -> (x < y?=w1570:bool)
              n627 = Multiply(x=w1558, y=w1574) -> (x*y=w1576:dbl)
              n628 = case shown="True" w1570 {
                tunnel: w1569 -> [w1586 w1589]
                tunnel: [w1586 w1590] -> w1562
                tunnel: w1557 -> [_ w1588]
                tunnel: [w1587 w1588] -> w1561
                tunnel: w1568 -> [w1587 _]
                frame False {
                }
                frame True {
                  n629 = local write "Trigger Offset(sec)"(w1588) -> ()
                  n630 = Bundle By Name(cluster=w1589, "Trigger Offset(sec)"=w1588) -> (w1590:T10)
                }
              }
              n631 = local read "FreeRun"() -> (w1565:bool)
              n632 = Negate(x=w1557) -> (-x=w1556:dbl)
              n633 = Greater?(x=w1556, y=w1561) -> (0:w1563:bool)
              n634 = case shown="True" w1563 {
                tunnel: w1562 -> [w1581 w1584]
                tunnel: [w1581 w1585] -> w1559
                tunnel: w1557 -> [_ w1583]
                tunnel: [w1582 w1583] -> w1560
                tunnel: w1561 -> [w1582 _]
                frame False {
                }
                frame True {
                  n635 = local write "Trigger Offset(sec)"(w1583) -> ()
                  n636 = Bundle By Name(cluster=w1584, "Trigger Offset(sec)"=w1583) -> (w1585:T10)
                }
              }
              n637 = Multiply(x=20.0 ("buffer/ms"), y=w1560) -> (x*y=w1577:dbl)
              n638 = Absolute Value(x=w1577) -> (abs(x)=w1579:dbl)
              n639 = Less Than 0?(x=w1577) -> (x < 0?=w1580:bool)
              n640 = Round Toward +Infinity(x=w1579) -> (ceil(x): smallest int >= x=w1578:dbl)
              n641 = case shown="False" w1580 {
                tunnel: w1578 -> [_ w1595]
                tunnel: [0 w1594] -> w1573
                tunnel: [2 1] -> w1566
                tunnel: w1576 -> [_ _]
                frame False {
                }
                frame True {
                  n642 = To Long Integer(number=w1595) -> (32bit integer=w1594:i32)
                }
              }
              n643 = Select(t=0, s=w1565, f=w1566) -> (s? t:f=w1564:i32)
              n644 = Bundle By Name(cluster=w1572, "prebuffer"=w1573, "nextbuffer"=w1566, "addbuffs"=w1564) -> (w1571:T16)
            }
          }
        }
        frame 18 {
          # "??????????????"
          # "trigger offset(second)"
          n645 = Unbundle By Name(w1604) -> ("Trigger Unit"=w1602:u32)
          n646 = Unbundle By Name(w1599) -> ("df"=w1598:dbl)
          n647 = Not Equal?(x=w1602, y=w1596) -> (x != y?=w1603:bool)
          n648 = case shown="True" w1603 {
            tunnel: w1599 -> [w1614 w1616]
            tunnel: [w1614 w1616] -> w1606
            tunnel: w1596 -> [_ w1615]
            frame False {
            }
            frame True {
              n649 = case shown="0, Default" w1615 {
                frame 0, Default {
                  # "dB"
                }
                frame 1 {
                  # "Voltage"
                }
              }
            }
          }
          n650 = case shown="True" "Snap" {
            tunnel: w1597 -> [_ w1612]
            tunnel: w1598 -> [_ w1609]
            frame False {
            }
            frame True {
              n651 = Array Max & Min(array=w1612) -> (max index (indices)=w1607:i32)  [unwired: 3 out]
              n652 = local write "Snap"(FALSE ("Snap")) -> ()
              n653 = Multiply(x=w1607, y=w1609) -> (x*y=w1611:dbl)
              n654 = Round Toward -Infinity(1:w1611) -> (0:w1608:dbl)
              n655 = property on="Spectrum graph" class="WFGraph (strict)"("Active Cursor"=u32 0, "Cursor.Cursor X"=w1608, "Cursor.Cursor Index"=w1607) -> ()  [unwired: 2 in, 2 out]
            }
          }
        }
        frame 19 {
          n656 = Unbundle By Name(w1623) -> ("FreeRun"=w1624:bool)
          n657 = Not Equal?(x=w1624, y=w1620) -> (x != y?=w1617:bool)
          n658 = case shown="True" w1617 {
            tunnel: w1620 -> [_ w1632]
            tunnel: w1619 -> [w1625 w1627]
            tunnel: [w1625 w1626] -> w1618
            frame False {
            }
            frame True {
              n659 = Unbundle By Name(w1627) -> ("nextbuffer"=w1631:i32)
              n660 = Not(x=w1632) -> (.not. x?=w1633:bool)
              n661 = property on="Triggered" class="Bool (strict)"("Visible"=w1633) -> ()  [unwired: 2 in, 2 out]
              n662 = local read "FreeRun"() -> (w1630:bool)
              n663 = Select(t=0, s=w1630, f=w1631) -> (s? t:f=w1628:i32)
              n664 = Bundle By Name(cluster=w1627, "addbuffs"=w1628) -> (w1626:T16)
            }
          }
        }
        frame Default {
          # "every time (if no event)"
          n665 = Unbundle By Name(w1644) -> ("Y-axis chg"=w1638:bool, "update"=w1639:bool, "acquire"=w1643:bool)
          n666 = Or(x=w1639, y=w1638) -> (x .or. y?=w1637:bool)
          n667 = And(x=w1642, y=w1643) -> (x .and. y?=w1634:bool)
          n668 = case shown="True" w1634 {
            tunnel: w1644 -> [w1670 w1687]
            tunnel: [w1670 w1686] -> w1636
            tunnel: w1645 -> [_ w1677]
            tunnel: w1640 -> [_ _]
            tunnel: w1642 -> [w1669 _]
            tunnel: w1641 -> [_ w1680]
            frame False {
              n669 = case shown="False" w1669 {
                frame False {
                  n670 = Square Root(x=-1.0) -> (sqrt(x)=w1671:dbl)
                  n671 = local write "dB"(w1671) -> ()
                  n672 = local write "Hz"(w1671) -> ()
                }
                frame True {
                }
              }
            }
            frame True {
              n673 = property on="Spectrum graph" class="WFGraph (strict)"("Active Cursor"=u32 0) -> ("Cursor.CursorMode"=w1678:u32)  [unwired: 2 in, 2 out]
              n674 = Unbundle By Name(w1687) -> ("df"=w1679:dbl, "window constants"=w1685:cluster{"eq noise BW":dbl, "coherent gain":dbl}, "db ref"=w1688:dbl)
              n675 = case shown="0" w1678 {
                tunnel: [w1690 w1695] -> w1682
                tunnel: w1679 -> [w1692 w1697]
                frame 0 {
                  n676 = property on="Spectrum graph" class="WFGraph (strict)"() -> ("Cursor.Cursor X"=w1689:dbl)  [unwired: 2 in, 2 out]
                  n677 = Divide(x=w1689, y=w1692) -> (x/y=w1693:dbl)
                  n678 = Round Toward +Infinity(x=w1693) -> (ceil(x): smallest int >= x=w1691:dbl)
                  n679 = Multiply(x=w1691, y=w1692) -> (x*y=w1690:dbl)
                }
                frame Default {
                  n680 = property on="Spectrum graph" class="WFGraph (strict)"("Active Cursor"=u32 0) -> ("Cursor.Cursor Index"=w1694:i32)  [unwired: 2 in, 2 out]
                  n681 = Multiply(x=w1694, y=w1697) -> (x*y=w1695:dbl)
                }
              }
              n682 = call <vilib>:"Power & Frequency Estimate.vi"("df"=w1679, "window constants"=w1685, "peak frequency (max)"=w1682, "Power Spectrum (V^2 rms)"=w1680) -> ("est power peak"=w1681:dbl, "est frequency peak"=w1684:dbl)  [unwired: 1 in, 1 out]
              "Hz" <- w1684
              n683 = Square Root(x=w1681) -> (sqrt(x)=w1674:dbl)
              n684 = call "CRYConversion dB-Lin.vi"("dB ref."=w1688, "Lin In"=w1674) -> ("Log Out"=w1675:dbl)  [unwired: 4 in, 3 out]
              "dB Est.Level" <- w1675
              n685 = Equal To 0?(x=w1677) -> (x = 0?=w1676:bool)
              n686 = Bundle By Name(cluster=w1687, "est freq"=w1684, "est power"=w1681) -> (w1686:T16)
              n687 = Select(t=w1675, s=w1676, f=w1674) -> (s? t:f=→"dB":dbl)
            }
          }
          n688 = case shown="True" w1637 {
            tunnel: w1640 -> [_ w1652]
            tunnel: w1636 -> [w1648 w1651]
            tunnel: [w1648 w1650] -> w1635
            frame False {
            }
            frame True {
              n689 = case shown="0, Default" w1652 {
                frame 0, Default {
                  n690 = local read "Y Unit"() -> (w1654:string)
                  n691 = Concatenate Strings("Amplitude [" ("string"), w1654, "]" ("string")) -> (w1656:string)
                  n692 = property on="Time graph" class="WFGraph (strict)"("YScale.NameLbl.Text"=w1656) -> ()  [unwired: 2 in, 2 out]
                }
                frame 1 {
                  n693 = local read "dB ref."() -> (w1661:dbl)
                  n694 = local read "Y-axis"() -> (w1662:u16)
                  n695 = local read "Y Unit"() -> (w1663:string)
                  n696 = case shown="0, Default" w1662 {
                    tunnel: [w1665 w1668] -> w1658
                    tunnel: w1661 -> [w1666 _]
                    tunnel: w1663 -> [w1664 w1668]
                    frame 0, Default {
                      n697 = Format Into String(format string="dB re %.p %s", w1666, w1664) -> (resulting string=w1665:string)  [unwired: 2 in, 1 out]
                    }
                    frame 1 {
                    }
                  }
                  n698 = Concatenate Strings("Amplitude [" ("string"), w1658, "]" ("string")) -> (w1657:string)
                  n699 = property on="Spectrum graph" class="WFGraph (strict)"("YScale.NameLbl.Text"=w1657) -> ()  [unwired: 2 in, 2 out]
                }
              }
              n700 = Bundle By Name(cluster=w1651, "Y-axis chg"=FALSE) -> (w1650:T16)
            }
          }
        }
      }
      n701 = Not(x=w759) -> (.not. x?=w758:bool)
    }
    n702 = Unbundle By Name(w269) -> ("acquire"=w249:bool)
    n703 = case shown="True" w249 {
      tunnel: w269 -> [w341 w468]
      tunnel: [w340 w453] -> w254
      tunnel: w241 -> [w335 w463]
      tunnel: [w349 w457] -> w263
      tunnel: w260 -> [w349 w456]
      tunnel: [w338 w455] -> w265
      tunnel: w262 -> [w338 w452]
      tunnel: [w339 w450] -> w264
      tunnel: w261 -> [w339 w401]
      tunnel: [w346 w447] -> w252
      tunnel: [w347 w446] -> w256
      tunnel: w268 -> [w343 _]
      tunnel: w236 -> [w348 w442]
      tunnel: [w348 w441] -> w259
      tunnel: w241 -> [_ w432]
      tunnel: [w332 w390] -> w232
      tunnel: w231 -> [w332 w389]
      frame False {
        n704 = Unbundle By Name(w335) -> ("Y-axis"=w334:u16)
        n705 = Wait (ms)(milliseconds to wait=u32 20) -> ()  [unwired: 1 out]
        n706 = Unbundle By Name(w341) -> ("db-pr factor"=w336:dbl, "df"=w333:dbl, "window constants"=w337:cluster{"eq noise BW":dbl, "coherent gain":dbl}, "update"=w345:bool)
        n707 = Or(x=w343, y=w345) -> (x .or. y?=w347:bool)
        n708 = Compound Arithmetic op=AND(invert w343, w345) -> (w344:bool)
        n709 = case shown="True" w344 {
          tunnel: [cluster{dbl, "df":dbl, "Spectrum":dbl[]} {0.0, "df"=0.0, "Spectrum"=[]} w370] -> w346
          tunnel: w338 -> [_ w362]
          tunnel: w333 -> [_ w364]
          tunnel: w337 -> [_ w366]
          tunnel: w336 -> [_ w365]
          tunnel: w334 -> [_ w363]
          frame False {
          }
          frame True {
            n710 = Equal To 0?(x=w363) -> (x = 0?=w368:bool)
            n711 = Boolean To (0,1)(Boolean=w368) -> (0, 1=w367:i16)
            n712 = call "CRYSpectrum Unit Conv dBref.vi"("window constants"=w366, "dB ref."=w365, "df"=w364, "display unit"=T15."Vrms", "log/linear"=w367, "Spectrum"=w362) -> ("Spectrum"=w361:dbl[])  [unwired: 2 in, 3 out]
            n713 = Bundle(0.0, "df"=w364, "Spectrum"=w361) -> (w370:cluster{dbl, "df":dbl, "Spectrum":dbl[]})  [unwired: 1 out]
          }
        }
        n714 = local read "Audio Driver"() -> (w331:u16)
        n715 = case shown="2" w331 {
          frame 2 {
            # "ASIO"
            n716 = local read "Rcv Idx"() -> (w351:u16)
            n717 = call "CRYCheck Main Receiver.vi"("Rcv Idx"=w351) -> ("Is Main?"=w352:bool)  [unwired: 10 in]
            n718 = local read "ASIO_Inited"() -> (w354:bool)
            n719 = local write "isMain"(w352) -> ()
            n720 = And(x=w354, y=w352) -> (x .and. y?=w353:bool)
            n721 = case shown="False" w353 {
              tunnel: w351 -> [_ w357]
              frame False {
                n722 = local write "Buf Cnt"(-1 ("Buf Cnt")) -> ()
              }
              frame True {
                n723 = local read "Asio OCI"() -> (w358:u32)
                n724 = call "CRYASIO Receive Data.vi"("Rcv Idx"=w357, "Limit"=w358, "Data Length"=2048, "Last Remain Buffer"=i32[] []) -> ()  [unwired: 5 in, 3 out]
              }
            }
          }
          frame 0, Default {
            # "MME/WDM"
          }
        }
        n725 = Bundle By Name(cluster=w341, "update"=FALSE ("Bundle Element")) -> (w340:T16)
      }
      frame True {
        w440 = FALSE ("Bundle Element")
        n726 = local read "Audio Driver"() -> (w375:u16)
        n727 = local read "initialized array"() -> (w393:i32[])
        n728 = Unbundle By Name(w463) -> ("n points"=w413:i32, "Averages"=w459:i32, "Weighting"=w458:u16, "Y-axis"=w433:u16, "Power/Complex"=w451:i32, "Time(sec)"=w415:dbl)
        n729 = local read "Sampling rate"() -> (w425:u32)
        n730 = Unbundle By Name(w468) -> ("buffers"=w418:i32, "addbuffs"=w412:i32, "trig level"=w430:i32, "halt acq"=w466:bool, "cal factor"=w377:dbl, "db-pr factor"=w460:dbl, "n avgd"=w444:i32, "points chg"=w398:bool, "update"=w422:bool, "Weight"=w392:cluster{dbl, dbl}[])
        n731 = case shown="0, Default" w375 {
          tunnel: [w517 u32 0 ("millisecond timer value")] -> w461
          tunnel: w415 -> [w516 _]
          frame 0, Default {
            n732 = Divide(x=w516, y=5.0) -> (x/y=w515:dbl)
            n733 = Wait (ms)(milliseconds to wait=w515) -> (millisecond timer value=w517:u32)
          }
          frame 2 {
          }
        }
        n734 = local read "Channel In"() -> (w372:u16)
        n735 = local read "Device In"() -> (w424:u32)
        n736 = local read "Bits"() -> (w423:u32)
        n737 = Add(x=w418, y=w412) -> (x+y=w417:i32)
        n738 = Boolean To (0,1)(Boolean=w422) -> (0, 1=w421:i16)
        n739 = local read "Sampling rate"() -> (w396:u32)
        n740 = Equal To 0?(x=w375) -> (x = 0?=w386:bool)
        n741 = Select(t=0.1 ("x"), s=w386, f=0.05 ("x")) -> (s? t:f=w385:dbl)
        n742 = Multiply(x=w415, y=w396) -> (x*y=w414:dbl)
        n743 = Multiply(x=w385, y=w396) -> (x*y=w395:dbl)
        n744 = To Long Integer(number=w395) -> (32bit integer=w394:i32)
        n745 = while {
          tunnel: w461 -> [_]
          tunnel: w423 -> [w534]
          tunnel: w425 -> [w535]
          tunnel: w424 -> [w536]
          tunnel: w417 -> [w538]
          tunnel: w466 -> [w529]
          shift-left: 0 -> [w542]
          shift-right: [w541] -> _
          tunnel: u8 0 ("OverHead") -> [w530]
          shift-left: i32[] [] -> [w544]
          shift-right: [w543] -> w388
          tunnel: w393 -> [w533]
          tunnel: 0.05 ("TimeRate") -> [w532]
          tunnel: 0.0 ("timeOut") -> [w531]
          tunnel: [w526] -> w434
          shift-right: [w521] -> w438
          shift-left: u8 0 ("OverHead") -> [w527]
          shift-right: [i16 0] -> _
          shift-left: w421 -> [w525]
          tunnel: w394 -> [w522]
          tunnel: w375 -> [w520]
          tunnel: w372 -> [w519]
          stop <- w539 continue-if-true
          n746 = case shown="2" w520 {
            tunnel: w544 -> [w552 w618]
            tunnel: [w550 w617] -> w543
            tunnel: w542 -> [w559 w616]
            tunnel: [w558 w615] -> w541
            tunnel: [w549 w614] -> w540
            tunnel: w538 -> [w557 w613]
            tunnel: w536 -> [_ w612]
            tunnel: w535 -> [_ w611]
            tunnel: w534 -> [_ w610]
            tunnel: w533 -> [_ w609]
            tunnel: w532 -> [_ w608]
            tunnel: w531 -> [_ w607]
            tunnel: w530 -> [_ w606]
            tunnel: w527 -> [w555 w595]
            tunnel: [FALSE w594] -> w526
            tunnel: w525 -> [_ w593]
            tunnel: w522 -> [w560 w592]
            tunnel: [w553 w589] -> w521
            tunnel: w519 -> [w548 _]
            frame 2 {
              # "ASIO"
              n747 = local read "Rcv Idx"() -> (w546:u16)
              n748 = call "CRYCheck Main Receiver.vi"("Rcv Idx"=w546) -> ("Is Main?"=w547:bool)  [unwired: 10 in]
              n749 = local read "ASIO_Inited"() -> (w561:bool)
              n750 = case shown="True" w561 {
                tunnel: w560 -> [w562 w571]
                tunnel: [0 ("Over Load") w570] -> w554
                tunnel: [w564 w569] -> w551
                tunnel: w548 -> [_ w566]
                tunnel: w547 -> [_ w567]
                tunnel: w546 -> [_ w568]
                frame False {
                  n751 = Initialize Array(0 ("element"), w562) -> (w564:i32[])
                }
                frame True {
                  n752 = case shown="True" w567 {
                    tunnel: w571 -> [w577 w585]
                    tunnel: [w576 w584] -> w570
                    tunnel: [w575 w583] -> w569
                    tunnel: w568 -> [w572 _]
                    tunnel: w566 -> [_ w581]
                    frame True {
                      n753 = local read "Remain Data"() -> (w578:i32[])
                      n754 = local read "Asio OCI"() -> (w574:u32)
                      n755 = call "CRYASIO Receive Data.vi"("Rcv Idx"=w572, "Limit"=w574, "Data Length"=w577, "Last Remain Buffer"=w578) -> ("Over Load"=w576:i32, "Data Out"=w575:i32[], "Remain Data"=w573:i32[])  [unwired: 5 in]
                      n756 = local write "Remain Data"(w573) -> ()
                      n757 = Array Size(array=w573) -> ()  [unwired: 1 out]
                    }
                    frame False {
                      n758 = local read "Remain Data"() -> (w586:i32[])
                      n759 = local read "Buf Cnt"() -> (w580:i32)
                      n760 = call "CRYASIO Receive Global Data.vi"("buf count"=w580, "Chn Idx"=w581, "Data Length"=w585, "Last Remain Buffer"=w586) -> ("Over Load"=w584:i32, "bufCount"=w579:i32, "Data Out"=w583:i32[], "Remain Data"=w582:i32[])  [unwired: 4 in]
                      n761 = local write "Buf Cnt"(w579) -> ()
                      n762 = local write "Remain Data"(w582) -> ()
                      n763 = Array Size(array=w582) -> ()  [unwired: 1 out]
                    }
                  }
                }
              }
              n764 = local write "isMain"(w547) -> ()
              n765 = local write "Real Time"(u8 9 ("Real Time")) -> ()
              n766 = Increment(x=w559) -> (x+1=w558:i32)
              n767 = Less?(x=w558, y=w557) -> (x < y?=w549:bool)
              n768 = Build Array (concatenate)(w552, w551) -> (w550:i32[])
              n769 = Add(x=w555, y=w554) -> (x+y=w553:i32)
            }
            frame 0, Default {
              (unwired) u8 1 ("StartFlag")
              # "MME/WDM"
              n770 = local read "start_flg"() -> (w587:u8)
              n771 = dll-call lib="D:/A_CRYSoundLab_Work/CRY6181/CRYSound.dll" fn="GVContinueRecord"("DeviceID"=w612, "nSampleFreq"=w611, "nChannels"=u32 2, "BitDepth"=w610, "TimeRate"=w608, "mode"=u32 0, "timeOut"=w607, "RecData"=w609, "StartFlag"=w587, "PauseFlag"=w606, "ChangeFlag"=w593, "taskID"="taskID") -> ("return type"=w588:u32, "nBufferUse"=w598:u32, "RealTime"=w602:u32, "RecData"=w604:i32[], "RecDataLen"=w601:u32, "OverHead"=w596:u8, "taskID"=w599:u32)  [unwired: 11 in, 8 out]
              n772 = To Unsigned Byte Integer(number=w602) -> (unsigned 8bit integer=→"Real Time":u8)
              n773 = local write "taskID"(w599) -> ()
              n774 = To Unsigned Byte Integer(number=w598) -> (unsigned 8bit integer=→"Buffer":u8)
              n775 = case shown="2" w588 {
                frame 0, Default {
                }
                frame 2 {
                  n776 = local write "start_flg"(u8 0 ("start_flg")) -> ()
                  n777 = local write "Start"(FALSE ("Start")) -> ()
                }
              }
              n778 = Equal To 0?(x=w601) -> (x = 0?=w605:bool)
              n779 = Add(x=w596, y=w595) -> (x+y=w589:i32)
              n780 = Not Equal To 0?(x=w588) -> (x != 0?=w594:bool)
              n781 = case shown="False" w605 {
                tunnel: w604 -> [w623 _]
                tunnel: w618 -> [w627 w630]
                tunnel: [w626 w630] -> w617
                tunnel: w616 -> [w625 w629]
                tunnel: [w624 w629] -> w615
                tunnel: w592 -> [w621 _]
                frame False {
                  n782 = Array Subset(array=w623, length=w621) -> (w622:i32[])  [unwired: 1 in]
                  n783 = Increment(x=w625) -> (x+1=w624:i32)
                  n784 = Build Array (concatenate)(w627, w622) -> (w626:i32[])
                }
                frame True {
                  n785 = Wait (ms)(milliseconds to wait=u32 21) -> ()  [unwired: 1 out]
                }
              }
              n786 = Less?(x=w615, y=w613) -> (x < y?=w614:bool)
            }
          }
          n787 = local read "Cancel"() -> (w537:bool)
          n788 = local read "Start"() -> (w524:bool)
          n789 = local read "OK"() -> (w528:bool)
          n790 = Compound Arithmetic op=AND(invert w529, w540, invert w537, invert w528, w524) -> (w539:bool)
        }
        n791 = To Long Integer(number=w414) -> (32bit integer=w408:i32)
        n792 = Greater Than 0?(x=w412) -> (x > 0?=w411:bool)
        n793 = Select(t=0 ("Output Element"), s=w398, f=w444) -> (s? t:f=w443:i32)
        n794 = local read "Channel In"() -> (w387:u16)
        n795 = local read "Audio Driver"() -> (w381:u16)
        n796 = local read "Channels"() -> (w380:u8)
        n797 = local read "Trigger Offset(sec)"() -> (w428:dbl)
        n798 = local read "Trigger Level"() -> (w406:dbl)
        n799 = Equal To 0?(x=w387) -> (x = 0?=w462:bool)
        n800 = local read "Trigger Unit"() -> (w404:u32)
        n801 = local read "FreeRun"() -> (w410:bool)
        n802 = case shown="2" w375 {
          tunnel: w411 -> [w478 w500]
          tunnel: w410 -> [w477 w499]
          tunnel: [w476 w496] -> w409
          tunnel: w408 -> [w475 w498]
          tunnel: w388 -> [w474 w497]
          frame 0, Default {
            # "WDM/MME"
            n803 = case shown="True" w478 {
              tunnel: w474 -> [w481 w492]
              tunnel: [w480 w492] -> w476
              tunnel: w477 -> [w482 _]
              tunnel: w475 -> [w479 w493]
              frame False {
                n804 = case shown="False" w482 {
                  tunnel: w481 -> [w489 w490]
                  tunnel: [w486 w490] -> w480
                  tunnel: w479 -> [w485 _]
                  frame False {
                    n805 = local read "rem buffer"() -> (w483:i32[])
                    n806 = Build Array (concatenate)(w483, w489) -> (w486:i32[])
                    n807 = Multiply(x=w485, y=2) -> (x*y=w488:i32)
                    n808 = Array Subset(array=w486, index=w488) -> (→"rem buffer":i32[])  [unwired: 1 in]
                  }
                  frame True {
                  }
                }
              }
              frame True {
                n809 = Multiply(x=w493, y=2) -> (x*y=w495:i32)
                n810 = Array Subset(array=w492, index=w495) -> (w491:i32[])  [unwired: 1 in]
                n811 = local write "rem buffer"(w491) -> ()
              }
            }
          }
          frame 2 {
            # "ASIO"
            n812 = case shown="False" w500 {
              tunnel: w497 -> [w503 w513]
              tunnel: [w502 w513] -> w496
              tunnel: w499 -> [w504 _]
              tunnel: w498 -> [w501 w511]
              frame False {
                n813 = case shown="False" w504 {
                  tunnel: w503 -> [w509 w510]
                  tunnel: [w508 w510] -> w502
                  tunnel: w501 -> [w505 _]
                  frame False {
                    n814 = local read "rem buffer"() -> (w507:i32[])
                    n815 = Build Array (concatenate)(w507, w509) -> (w508:i32[])
                    n816 = Array Subset(array=w508, index=w505) -> (w506:i32[])  [unwired: 1 in]
                    n817 = local write "rem buffer"(w506) -> ()
                  }
                  frame True {
                  }
                }
              }
              frame True {
                n818 = Array Subset(array=w513, index=w511) -> (w512:i32[])  [unwired: 1 in]
                n819 = local write "rem buffer"(w512) -> ()
              }
            }
          }
        }
        n820 = Equal To 0?(x=w381) -> (x = 0?=w382:bool)
        n821 = local read "dT(sec)"() -> (w420:dbl)
        n822 = call "CRYData throw-away decide.vi"("Maximum % processed (20%)"=100.0, "Iteration"=w443) -> ("Suppress processing"=w429:bool)  [unwired: 1 in, 8 out]
        n823 = Select(t=w380, s=w382, f=u8 1) -> (s? t:f=w378:u8)
        n824 = call "CRYChannel separate buffer array.vi"("N channels"=w378, "Buffer array in"=w409) -> ("First right channel"=w464:i32[], "First left channel"=w465:i32[])  [unwired: 8 out]
        n825 = Select(t=w465, s=w462, f=w464) -> (s? t:f=w376:i32[])
        n826 = Multiply(x=w376, y=w377) -> (x*y=w374:dbl[])
        n827 = Array Max & Min(array=w401) -> (max value=w405:dbl)  [unwired: 3 out]
        n828 = Equal To 0?(x=w404) -> (x = 0?=w399:bool)
        n829 = Less Or Equal?(x=w406, y=w405) -> (x <= y?=w407:bool)
        n830 = case shown="0, Default" w375 {
          tunnel: w374 -> [w470 w473]
          tunnel: [w470 w471] -> w373
          frame 0, Default {
          }
          frame 2 {
            n831 = Divide(x=w473, y=512.0) -> (x/y=w471:dbl[])
          }
        }
        n832 = Multiply(x=w428, y=1000.0) -> (x*y=w426:dbl)
        n833 = Or(x=w398, y=w399) -> (x .or. y?=w397:bool)
        n834 = Compound Arithmetic op=AND(w399, w407) -> (w400:bool)
        n835 = call "CRYTrigger advanced.vi"("N sample"=w408, "N points"=w413, "Slope"="Slope", "Signal"=w373, "Pretrigger ms"=w426, "Trigger level (counts)"=w430, "dt"=w420, "Free run"=w410, "Reset buffer"=w397) -> ("Triggered signal"=w391:dbl[], "Triggered"=w403:bool)  [unwired: 5 out]
        n836 = Or(x=w403, y=w400) -> (x .or. y?=w402:bool)
        "Triggered" <- w402
        n837 = Compound Arithmetic op=OR(invert w402, w434, w429) -> (w449:bool)
        n838 = Not(x=w466) -> (.not. x?=w467:bool)
        n839 = Bundle By Name(cluster=w468, "acquire"=w467, "halt acq"=w440, "points chg"=w440, "update"=w440, "addbuffs"=0) -> (w454:T16)
        n840 = case shown="False" w449 {
          tunnel: w391 -> [w631 _]
          tunnel: w377 -> [w664 _]
          tunnel: w460 -> [w663 _]
          tunnel: w459 -> [w632 _]
          tunnel: w458 -> [w657 _]
          tunnel: [w662 w740] -> w457
          tunnel: w456 -> [w646 w740]
          tunnel: w433 -> [w644 _]
          tunnel: [w634 w739] -> w455
          tunnel: w454 -> [w659 w736]
          tunnel: [w658 w734] -> w453
          tunnel: w452 -> [_ w739]
          tunnel: w420 -> [w643 _]
          tunnel: w451 -> [w655 _]
          tunnel: [w638 w732] -> w450
          tunnel: w443 -> [w654 w735]
          tunnel: w401 -> [_ w732]
          tunnel: [w639 cluster{dbl, "df":dbl, "Spectrum":dbl[]} {0.0, "df"=0.0, "Spectrum"=[]}] -> w447
          tunnel: [TRUE FALSE] -> w446
          tunnel: w442 -> [w652 w733]
          tunnel: [w651 w733] -> w441
          tunnel: w438 -> [w650 _]
          tunnel: w432 -> [_ _]
          tunnel: w402 -> [_ _]
          tunnel: w392 -> [w633 _]
          tunnel: [w631 w731] -> w390
          tunnel: w389 -> [_ w731]
          frame False {
            n841 = Not Equal To 0?(x=w650) -> (x != 0?=w642:bool)
            "Overload" <- w642
            n842 = Equal To 0?(x=w654) -> (x = 0?=w653:bool)
            n843 = Multiply(x=w631, y=w664) -> ()  [unwired: 1 out]
            n844 = Greater Than 0?(x=w657) -> (x > 0?=w656:bool)
            n845 = property on="Overload" class="Bool (strict)"("闪烁"=w642) -> ()  [unwired: 2 in, 2 out]
            n846 = Increment(x=w654) -> (x+1=w635:i32)
            n847 = case shown="0, Default" w655 {
              tunnel: w631 -> [w698 w711]
              tunnel: w632 -> [w697 w707]
              tunnel: w656 -> [_ _]
              tunnel: [w696 w708] -> w660
              tunnel: "Window" -> [w695 w710]
              tunnel: w643 -> [w694 w709]
              tunnel: [w690 w704] -> w640
              tunnel: w653 -> [w693 w706]
              tunnel: [w692 w699] -> w634
              tunnel: w633 -> [w691 w702]
              frame 0, Default {
                # "Power"
                n848 = call "CRYFFT CRYSoundLab.vi"("dt"=w694, "Window"=w695, "Time series"=w698) -> ("window constants"=w696:cluster{"eq noise BW":dbl, "coherent gain":dbl}, "df"=w690:dbl, "Power Spectrum (V^2 rms)"=w688:dbl[])  [unwired: 6 out]
                n849 = To Double Precision Complex(1:w688) -> (0:w687:cdb[])
                n850 = call "CRYCalc Weighting.vi"("Weight"=w691, "df"=w690, "Complex FFT (Vrms)"=w687) -> ("Weighted Com"=w686:cdb[])  [unwired: 8 in]
                n851 = Complex To Re/Im(x + iy=w686) -> (x=w685:dbl[])  [unwired: 1 out]
                n852 = call "CRYCurve averaging real-time fft.vi"("Initialize (F)"=w693, "Exponential averaging? (F=linear)"=TRUE, "Number of averages (no change)"=w697, "Input curve"=w685) -> ("Averaged curve"=w692:dbl[])  [unwired: 7 out]
              }
              frame 1 {
                # "Complex"
                n853 = call "CRYFFT CRYSoundLab complex.vi"("dt"=w709, "Window"=w710, "Time series"=w711) -> ("window constants"=w708:cluster{"eq noise BW":dbl, "coherent gain":dbl}, "df"=w704:dbl, "Complex FFT (Vrms)"=w705:cdb[])  [unwired: 6 out]
                n854 = call "CRYCalc Weighting.vi"("Weight"=w702, "df"=w704, "Complex FFT (Vrms)"=w705) -> ("Weighted Com"=w703:cdb[])  [unwired: 8 in]
                n855 = call "CRYCurve complex averaging real-time fft.vi"("Initialize (F)"=w706, "Exponential averaging? (F=linear)"=TRUE, "Number of averages (no change)"=w707, "Input curve, complex"=w703) -> ("Averaged curve"=w700:dbl[])  [unwired: 7 out]
                n856 = Complex To Polar(r * e^(i*theta)=w700) -> ()  [unwired: 2 out]
                n857 = Complex To Re/Im(x + iy=w700) -> (x=w699:dbl[])  [unwired: 1 out]
              }
            }
            n858 = Equal To 0?(x=w644) -> (x = 0?=w665:bool)
            n859 = Boolean To (0,1)(Boolean=w665) -> (0, 1=w661:i16)
            n860 = Not(x=w653) -> (.not. x?=w637:bool)
            n861 = local read "A/M/M"() -> (w645:i32)
            n862 = call "CRYSpectrum Unit Conv dBref.vi"("window constants"=w660, "dB ref."=w663, "df"=w640, "display unit"=T15."Vrms", "log/linear"=w661, "Spectrum"=w634) -> ("Spectrum"=w636:dbl[])  [unwired: 2 in, 3 out]
            n863 = case shown="True" w637 {
              tunnel: w646 -> [_ w717]
              tunnel: [w712 w714] -> w638
              tunnel: [w712 w714] -> w662
              tunnel: w636 -> [w712 w716]
              tunnel: w645 -> [_ w715]
              tunnel: w635 -> [_ w713]
              frame False {
              }
              frame True {
                n864 = case shown="0, Default" w715 {
                  tunnel: w717 -> [_ w721 w727]
                  tunnel: [w718 w720 w725] -> w714
                  tunnel: w716 -> [w718 w719 w726]
                  tunnel: w713 -> [_ _ _]
                  frame 0, Default {
                  }
                  frame 1 {
                    n865 = for {
                      tunnel: w721 -> [w724] mode=indexing
                      tunnel: [w723] -> w720 mode=indexing
                      tunnel: w719 -> [w722] mode=indexing
                      n866 = Max & Min(x=w724, y=w722) -> (max(x,y)=w723:dbl)  [unwired: 1 out]
                    }
                  }
                  frame 2 {
                    n867 = for {
                      tunnel: w727 -> [w730] mode=indexing
                      tunnel: w726 -> [w729] mode=indexing
                      tunnel: [w728] -> w725 mode=indexing
                      n868 = Max & Min(x=w730, y=w729) -> (min(x,y)=w728:dbl)  [unwired: 1 out]
                    }
                  }
                }
              }
            }
            n869 = case shown="3" w652 {
              tunnel: w644 -> [_ w677]
              frame Default {
              }
              frame 3 {
                n870 = stacked-sequence {
                  tunnel: w677 -> [_ w679 w681]
                  frame #0 {
                    n871 = disable-structure shown="Disabled" {
                      frame Disabled {
                        n872 = property on="Spectrum graph" class="WFGraph (strict)"("Y标尺.标尺调节"=u8 0 ("Write Attribute")) -> ()  [unwired: 2 in, 2 out]
                      }
                      frame Enabled {
                      }
                    }
                  }
                  frame #1 {
                    n873 = case shown="0" w679 {
                      frame 0 {
                        n874 = Wait (ms)(milliseconds to wait=u32 5) -> ()  [unwired: 1 out]
                      }
                      frame Default {
                      }
                    }
                  }
                  frame #2 {
                    n875 = case shown="0" w681 {
                      frame 0 {
                        n876 = disable-structure shown="Disabled" {
                          frame Disabled {
                            n877 = property on="Spectrum graph" class="WFGraph (strict)"() -> ("Y标尺.范围:最大值"=w683:dbl)  [unwired: 2 in, 2 out]
                            n878 = Add(x=w683, y=10.0) -> (x+y=w682:dbl)
                            n879 = property on="Spectrum graph" class="WFGraph (strict)"("Y标尺.范围:最大值"=w682) -> ()  [unwired: 2 in, 2 out]
                          }
                          frame Enabled {
                          }
                        }
                      }
                      frame Default {
                      }
                    }
                  }
                }
              }
            }
            n880 = Increment(x=w652) -> (x+1=w651:i32)
            n881 = Bundle By Name(cluster=w659, "df"=w640, "window constants"=w660, "n avgd"=w635) -> (w658:T16)
            n882 = local read "Mode"() -> (w647:u32)
            n883 = case shown="0, Default" w647 {
              tunnel: w638 -> [_ w674]
              tunnel: w631 -> [w667 _]
              tunnel: w640 -> [_ w675]
              frame 0, Default {
                n884 = stacked-sequence {
                  tunnel: w667 -> [w668 _]
                  frame #0 {
                    n885 = local read "dT(sec)"() -> (w670:dbl)
                    n886 = Bundle(0.0, "dT(sec)"=w670, "Triggered signal"=w668) -> (→"Time graph":T7)  [unwired: 1 out]
                  }
                  frame #1 {
                    n887 = control-ref of="Time graph"() -> (w673:refnum<vi>)
                    n888 = call "CRYPaint WaterMark.vi"("Type"="Small", "Graph Ref"=w673) -> ()  [unwired: 10 in]
                  }
                }
              }
              frame 1 {
                n889 = Bundle(0.0, "df"=w675, "Spectrum"=w674) -> ()  [unwired: 2 out]
              }
            }
            n890 = Bundle(0.0, "df"=w640, "Spectrum"=w638) -> (w639:cluster{dbl, "df":dbl, "Spectrum":dbl[]})  [unwired: 1 out]
          }
          frame True {
            n891 = Bundle By Name(cluster=w736, "n avgd"=w735) -> (w734:T16)
          }
        }
      }
    }
    n892 = local read "Mode"() -> (w235:u32)
    n893 = case shown="0, Default" w235 {
      tunnel: [w289 w300] -> w233
      tunnel: [w288 w299] -> w234
      frame 0, Default {
        n894 = property on="Time graph" class="WFGraph (strict)"() -> ("CrsrList"=w292:T20)  [unwired: 2 in, 2 out]
        n895 = Index Array(array=w292, index #1=1 ("index"), index #2=0 ("index")) -> (element #1=w293:T21, element #2=w296:T21)
        n896 = Unbundle By Name(w293) -> ("Position.Y"=w291:dbl, "Position.X"=w298:dbl)
        n897 = Unbundle By Name(w296) -> ("Position.X"=w297:dbl, "Position.Y"=w290:dbl)
        n898 = Subtract(x=w291, y=w290) -> (x-y=w289:dbl)
        n899 = Subtract(x=w298, y=w297) -> (x-y=w288:dbl)
      }
      frame 1 {
        n900 = property on="Spectrum graph" class="WFGraph (strict)"() -> ("CrsrList"=w301:T20)  [unwired: 2 in, 2 out]
        n901 = Index Array(array=w301, index #1=1 ("index"), index #2=0 ("index")) -> (element #1=w304:T21, element #2=w307:T21)
        n902 = Unbundle By Name(w304) -> ("Position.Y"=w303:dbl, "Position.X"=w309:dbl)
        n903 = Unbundle By Name(w307) -> ("Position.X"=w308:dbl, "Position.Y"=w302:dbl)
        n904 = Subtract(x=w303, y=w302) -> (x-y=w300:dbl)
        n905 = Subtract(x=w309, y=w308) -> (x-y=w299:dbl)
      }
    }
    n906 = local write "delta_X"(w234) -> ()
    n907 = local write "delta_Y"(w233) -> ()
    n908 = Unbundle By Name(w254) -> ("autoscale"=w255:bool)
    n909 = Unbundle By Name(w241) -> ("Y-axis"=w257:u16)
    n910 = case shown="True" w256 {
      tunnel: w252 -> [_ w315]
      tunnel: w255 -> [_ w314]
      tunnel: w257 -> [_ w313]
      tunnel: w254 -> [w310 w312]
      tunnel: [w310 w311] -> w253
      frame False {
      }
      frame True {
        n911 = stacked-sequence {
          tunnel: w315 -> [w316 _]
          tunnel: w314 -> [_ _]
          tunnel: w313 -> [_ w320]
          tunnel: w312 -> [_ w319]
          tunnel: [_ w318] -> w311
          frame #0 {
            "Spectrum graph" <- w316
          }
          frame #1 {
            n912 = stacked-sequence {
              tunnel: w320 -> [_ w323 w325]
              frame #0 {
                n913 = control-ref of="Spectrum graph"() -> (w322:refnum<vi>)
                n914 = call "CRYPaint WaterMark.vi"("Type"="Small", "Graph Ref"=w322) -> ()  [unwired: 10 in]
              }
              frame #1 {
                n915 = case shown="0" w323 {
                  frame 0 {
                    n916 = Wait (ms)(milliseconds to wait=u32 5) -> ()  [unwired: 1 out]
                  }
                  frame Default {
                  }
                }
              }
              frame #2 {
                n917 = disable-structure shown="Disabled" {
                  disable-tunnel: w325 -> [w326 _]
                  frame Disabled {
                    n918 = case shown="0" w326 {
                      frame 0 {
                        n919 = disable-structure shown="Disabled" {
                          frame Disabled {
                            n920 = property on="Spectrum graph" class="WFGraph (strict)"() -> ("Y标尺.范围:最大值"=w328:dbl)  [unwired: 2 in, 2 out]
                            n921 = Add(x=w328, y=10.0) -> (x+y=w327:dbl)
                            n922 = property on="Spectrum graph" class="WFGraph (strict)"("Y标尺.范围:最大值"=w327) -> ()  [unwired: 2 in, 2 out]
                          }
                          frame Enabled {
                          }
                        }
                      }
                      frame Default {
                      }
                    }
                  }
                  frame Enabled {
                  }
                }
              }
            }
            n923 = Bundle By Name(cluster=w319, "autoscale"=FALSE ("Bundle Element")) -> (w318:T16)
          }
        }
      }
    }
    n924 = stacked-sequence {
      tunnel: ["cont loop"] -> w258
      tunnel: w254 -> [_]
      frame #0 {
      }
    }
  }
  n925 = stacked-sequence {
    tunnel: w4 -> [_ _ _ w1766 _]
    tunnel: w1 -> [_ _ _ w1760 _]
    frame #0 {
      w1702 = u32 0 ("nSampleFreq")
      n926 = local read "Device In"() -> (w1704:u32)
      n927 = local read "taskID"() -> (w1705:u32)
      n928 = local read "Rcv Idx"() -> (w1698:u16)
      n929 = local read "isMain"() -> (w1699:bool)
      n930 = local read "Audio Driver"() -> (w1700:u16)
      n931 = call "CRYClear Main Receiver Array.vi"("isMain"=w1699, "Rcv Idx"=w1698) -> ()  [unwired: 10 in]
      n932 = dll-call lib="D:/A_CRYSoundLab_Work/CRY6181/CRYSound.dll" fn="GVContinueRecord"("DeviceID"=w1704, "nSampleFreq"=w1702, "nChannels"=w1702, "BitDepth"=w1702, "TimeRate"=w1702, "mode"=w1702, "nBufferUse"=w1702, "RealTime"=w1702, "timeOut"=w1702, "RecData"=i32[] [], "RecDataLen"=w1702, "OverHead"=w1702, "StartFlag"=u8 0, "PauseFlag"=w1702, "ChangeFlag"=w1702, "taskID"=w1705) -> ()  [unwired: 10 in, 12 out]
      n933 = case shown="2" w1700 {
        frame 2 {
          n934 = local read "ASIO_Inited"() -> (w1706:bool)
          n935 = case shown="True" w1706 {
            frame False {
            }
            frame True {
              n936 = local read "Channel In"() -> (w1707:u16)
              n937 = local read "Asio OCI"() -> (w1708:u32)
              n938 = local write "ASIO_Inited"(FALSE ("ASIO_Inited")) -> ()
              n939 = call "CRYASIO Close Cur Channel & Dev.vi"("Limit"=w1708, "isInput?"=TRUE, "Channel Out"=w1707) -> ()  [unwired: 9 in]
            }
          }
        }
        frame 0, Default {
        }
      }
    }
    frame #1 {
      n940 = local read "Trigger Offset(sec)"() -> (w1729:dbl)
      n941 = local read "Power/Complex"() -> (w1739:i32)
      n942 = local read "Trigger Path"() -> (w1734:u16)
      n943 = local read "Trigger Level"() -> (w1728:dbl)
      n944 = local read "Trigger Unit"() -> (w1730:u32)
      n945 = local read "CalSpectrum"() -> (w1726:bool)
      n946 = property on="Weighting" class="Ring (strict)"() -> ("RingText.Text"=w1719:string)  [unwired: 2 in, 2 out]
      n947 = property on="Signal Path" class="Ring (strict)"() -> ("RingText.Text"=w1720:string)  [unwired: 2 in, 2 out]
      n948 = local read "Channel In"() -> (w1721:u16)
      n949 = property on="Y-axis" class="Ring (strict)"() -> ("RingText.Text"=w1717:string)  [unwired: 2 in, 2 out]
      n950 = global read "CRYMisc vis settings global.vi" "Rcv Index Array"() -> (w1713:T23)
      n951 = local read "Averages"() -> (w1737:i32)
      n952 = local read "Time(sec)"() -> (w1740:dbl)
      n953 = local read "FreeRun"() -> (w1727:bool)
      n954 = local read "Window"() -> (w1741:u16)
      n955 = local read "n points"() -> (w1735:i32)
      n956 = local read "Lin/Exp"() -> (w1736:i32)
      n957 = local read "Correct"() -> (w1733:bool)
      n958 = local read "A/M/M"() -> (w1732:i32)
      n959 = local read "Mode"() -> (w1738:u32)
      n960 = local read "Slope"() -> (w1731:u32)
      n961 = local read "Rcv Idx"() -> (w1711:u16)
      n962 = for {
        tunnel: w1713 -> [w1745] mode=indexing
        tunnel: [w1744] -> w1712 mode=indexing
        n963 = Unbundle By Name(w1745) -> ("Rcv Idx"=w1744:i32)
      }
      n964 = property on="Signal Path" class="Ring (strict)"() -> ("RingText.Text"=→"Selected Signal Path":string)  [unwired: 2 in, 2 out]
      n965 = global read "CRYMisc vis settings global.vi" "Scope-FFT settings"() -> (w1718:T12)
      n966 = Bundle By Name(cluster=w1718, "window"=w1741, "n avgs"=w1737, "lin/exp avg"=w1736, "pwr/cplx avg"=w1739, "time (ms)"=w1740, "fft lines"=w1735, "scope/fft mode"=w1738, "channel"=w1721, "trig. channel"=w1734, "Applay Correction"=w1733, "Time Display"="", "Freq. Weighting"=w1719, "Ave/Max/Min"=w1732, "Trigger Level"=w1728, "Trigger Unit"=w1730, "Trigger Time Offset"=w1729, "Trigger Slope"=w1731, "Trigger/Free Run"=w1727, "continuous"=FALSE, "Spectrum Display"="", "Calc FFT"=w1726, "Y-axis"=w1717, "Signal Type"=w1720) -> (w1742:T12)
      n967 = Search 1D Array(1D array=w1712, element=w1711) -> (index of element=w1715:i32)  [unwired: 1 in]
      n968 = call "CRYFlatten Scope-FFT.vi"("Scope-FFT settings"=w1742) -> ("Flat Scope-FFT settings"=→"scope-fft setup Out":string)  [unwired: 10 out]
      n969 = Delete From Array(array=w1713, index=w1715) -> (array with subset deleted=w1714:T23)  [unwired: 1 in, 1 out]
      n970 = local read "Cancel"() -> (w1722:bool)
      "Canceled" <- w1722
      n971 = case shown="False" w1722 {
        tunnel: w1742 -> [w1746 _]
        frame False {
          n972 = flat-sequence {
            tunnel: w1746 -> [w1747]
            frame #0 {
              n973 = global write "CRYMisc vis settings global.vi" "Scope-FFT settings"(w1747) -> ()
            }
            frame #1 {
              n974 = local read "Manual"() -> (w1748:bool)
              n975 = case shown="False" w1748 {
                frame False {
                  n976 = call "CRYSave Virtual Data.vi"() -> ()  [unwired: 1 in, 11 out]
                }
                frame True {
                }
              }
            }
          }
        }
        frame True {
        }
      }
      n977 = global write "CRYMisc vis settings global.vi" "Rcv Index Array"(w1714) -> ()
    }
    frame #2 {
      w1750 = FALSE ("Cancel")
      n978 = local write "OK"(w1750) -> ()
      n979 = local write "Cancel"(w1750) -> ()
      n980 = local write "Manual"(TRUE ("Manual")) -> ()
    }
    frame #3 {
      n981 = Unbundle By Name(w1766) -> ("db ref"=w1761:dbl, "df"=w1758:dbl)
      n982 = global read "CRYMisc vis settings global.vi" "CloseAll Event"() -> (w1765:bool)
      n983 = local read "Menu"() -> (w1763:bool)
      n984 = case shown="True" "close at end" {
        frame False {
        }
        frame True {
          n985 = property class="VI"("前面板窗口:打开"=FALSE ("Front Panel Window:Open")) -> ()  [unwired: 2 in, 2 out]
        }
      }
      n986 = Not(x=w1765) -> (.not. x?=w1764:bool)
      n987 = And(x=w1763, y=w1764) -> (x .and. y?=w1762:bool)
      n988 = case shown="True" w1762 {
        frame False {
        }
        frame True {
          n989 = local read "VI nID"() -> (w1768:i32)
          n990 = call "CRYOperator Process.vi"("VI ID"=w1768, "sAction"="Close", "sOperator Type"="OPERATOR_OSCILLOSCOPE" ("sAction")) -> ()  [unwired: 8 in, 1 out]
        }
      }
      n991 = local read "Sampling rate"() -> (w1754:u32)
      n992 = local read "Max Level"() -> (w1751:dbl)
      n993 = local read "Y-axis"() -> (w1755:u16)
      n994 = local read "Y Unit"() -> (w1757:string)
      n995 = To Double Precision Float(number=w1754) -> (double precision float=w1753:dbl)
      n996 = Bundle By Name(cluster=T22 {"Fs"=0.0, "df"=0.0, "db ref"=0.0, "X data"=1, "Y data"=0, "Y Unit"="", "Y"=[], "Max Level"=0.0}, "Fs"=w1753, "df"=w1758, "db ref"=w1761, "X data"=u16 1 ("X axis"), "Y data"=w1755, "Y Unit"=w1757, "Y"=w1760, "Max Level"=w1751) -> (→"Data cluster":T22)
    }
    frame #4 {
      n997 = local write "StateOut"(TRUE ("StateOut")) -> ()
    }
  }
